vi "StorePAQ.vi"(6 "AverageAction IN":T2, 8 "error in (no error)":errorcluster, 9 "Level":T1, 10 "StoreDatagram":T3 {"Time" format="%#.2f"; "status" format="%x"; "min" format="%.2f"; "max" format="%.2f"; "data" format="%.2f"}, 11 "FAMM in":refnum<class "FAMM.lvclass">) -> (0 "error out":errorcluster, 2 "Next_Level":T2, 3 "FAMM out":refnum<class "FAMM.lvclass">)   [LabVIEW 2020, in "Sgraph_lib_V1.lvlib" / "FAMM.lvclass"]
doc: "Store one element to the PAQ memory"
uses:
  FAMM.lvclass
  controls/MemStoreDatagram.ctl
  controls/typedef_AverageAction.ctl
  controls/typedef_Level.ctl
  FAMM.lvclass/FAMM.ctl
  PAQ-memory.lvclass
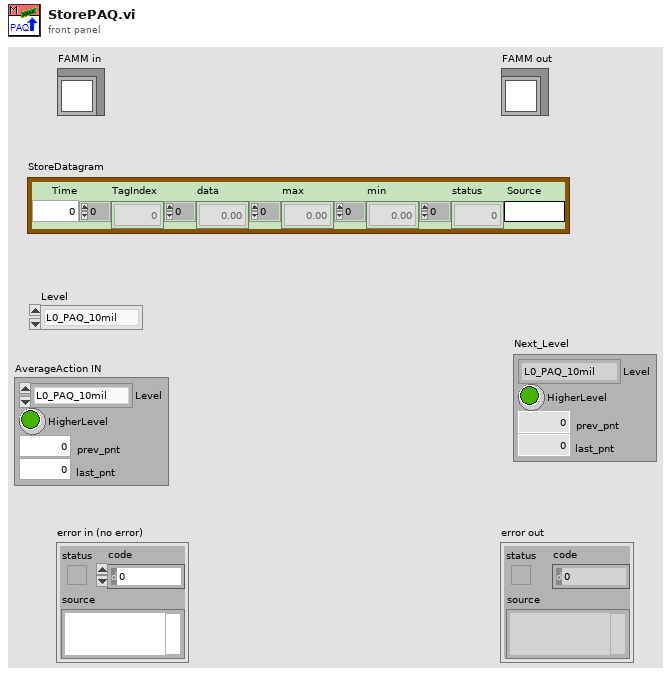
[diagram p1: front panel]
types:
  T1 = typedef "Sgraph_lib_V1.lvlib/FAMM.lvclass/typedef_Level.ctl" = enum16{"L0_PAQ_10mil", "L0_PAQ_100mil", "L1_PAQ_100mil", "L2_PAQ_1sec", "L3_PAQ_10sec", "L4_PAQ_1min", "L5_PAQ_10min", "L6_PAQ_2hr", "L7_PAQ_1day", "L8_PAQ_1wk", "L1_PAQ_1sec", "L2_PAQ_10sec", "L3_PAQ_1min", "L4_PAQ_10min", "L5_PAQ_2hr", "L6_PAQ_1day", "L7_PAQ_1wk", "L0_PAQ_1sec", "L1_PAQ_10sec", "L2_PAQ_1min", "L3_PAQ_10min", "L4_PAQ_2hr", "L5_PAQ_1day", "L6_PAQ_1wk", "L0_PAQ_10sec", "L1_PAQ_1min", "L2_PAQ_10min", "L3_PAQ_2hr", "L4_PAQ_1day", "L5_PAQ_1wk"}
  T2 = typedef "Sgraph_lib_V1.lvlib/FAMM.lvclass/typedef_AverageAction.ctl" = cluster{"Level":T1, "HigherLevel":bool, "prev_pnt":i32, "last_pnt":i32}
  T3 = typedef "Sgraph_lib_V1.lvlib/FAMM.lvclass/MemStoreDatagram.ctl" = cluster{"Time":dbl, "TagIndex":i32[], "data":dbl[], "max":dbl[], "min":dbl[], "status":u32[], "Source":string}
  T4 = cluster{"TAGs":i32[], "prev_pnt":i32, "last_pnt":i32}
  T5 = typedef "Sgraph_lib_V1.lvlib/FAMM.lvclass/FAMM-attributes.ctl" = cluster{"FAMM_PAQ_Layers":i32, "FAMM_PAQ_resolution":dbl, "PAQ_TAGs":string[], "WAQ_TAGs":string[], "EAQ_TAGs":string[], "All_TAGs":string[], "PAQtagProps":T6[], "WAQtagProps":T6[], "EAQtagProps":T6[], "DBAL_class":refnum<data-value>, "PAQ_memory":refnum<data-value>[], "PAQupdates":timestamp[], "FAMM_Size":cluster{"other":i32, "1day":i32, "1week":i32}, "DatabaseFileExtention":string, "DatabaseSaveRate":dbl, "Database_path":path, "DBAL-Queue":refnum<queue>, "OS_name":string, "ini-file":string, "data-retention(days)":dbl}
  T6 = typedef "Sgraph_lib_V1.lvlib/typedef_com_TagProp.ctl" = cluster{"Description":string, "EngUnits":string, "RangeH":dbl, "RangeL":dbl, "Resolution":i32, "Obsolete":bool, "ChangeDate":timestamp, "ChangeSource":string, "ChangeReason":string, "TagFunc":u32}
  T7 = cluster{"Time":dbl, "data":dbl[], "max":dbl[], "min":dbl[], "status":u32[]}
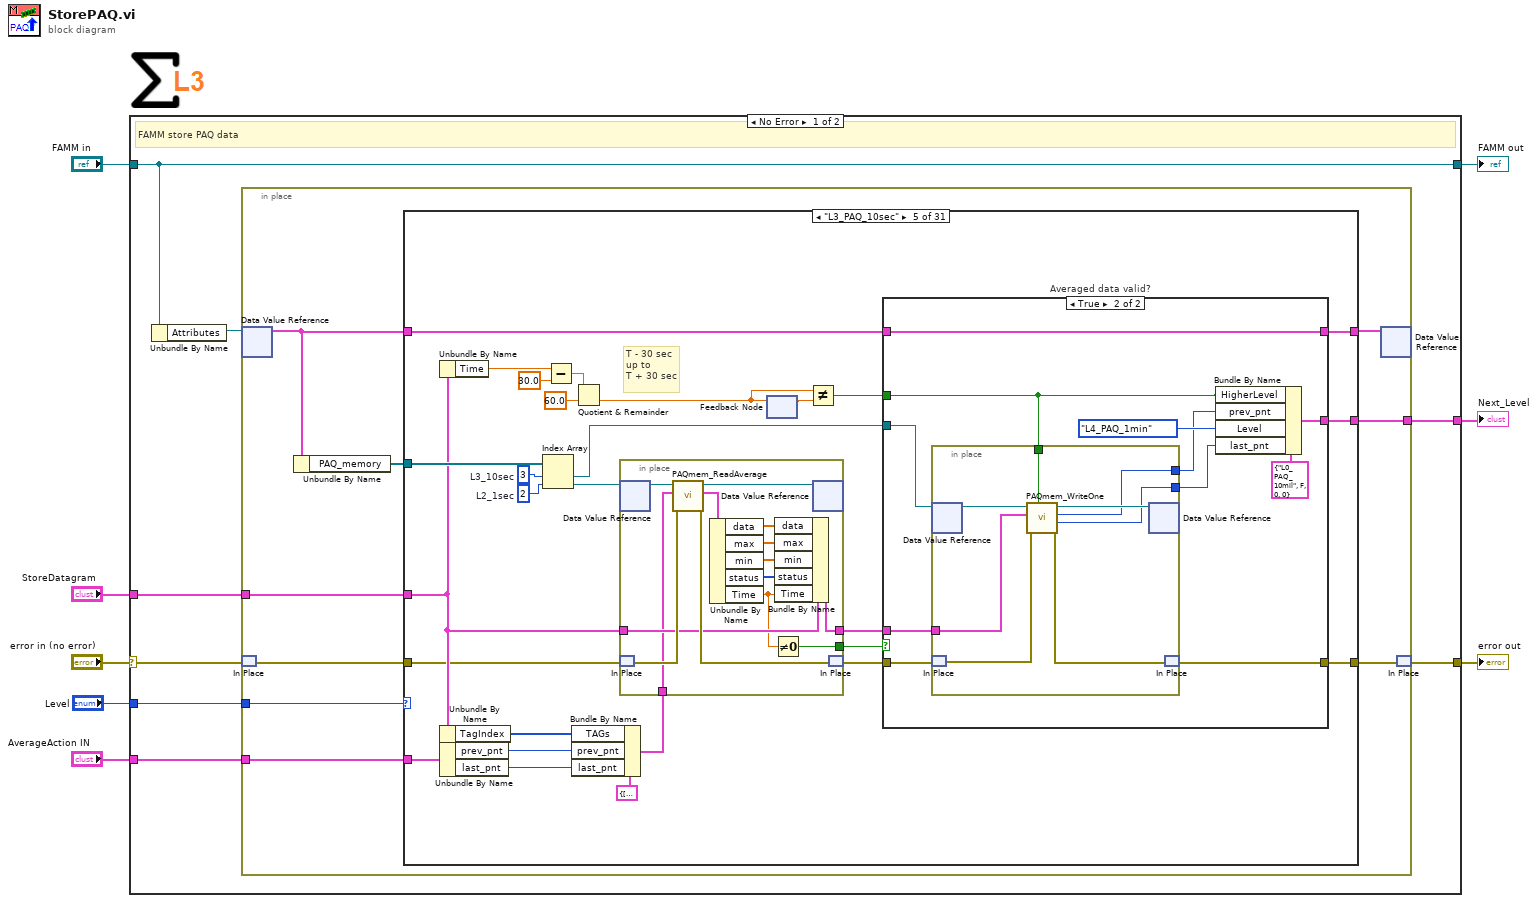
[diagram p0: block diagram]
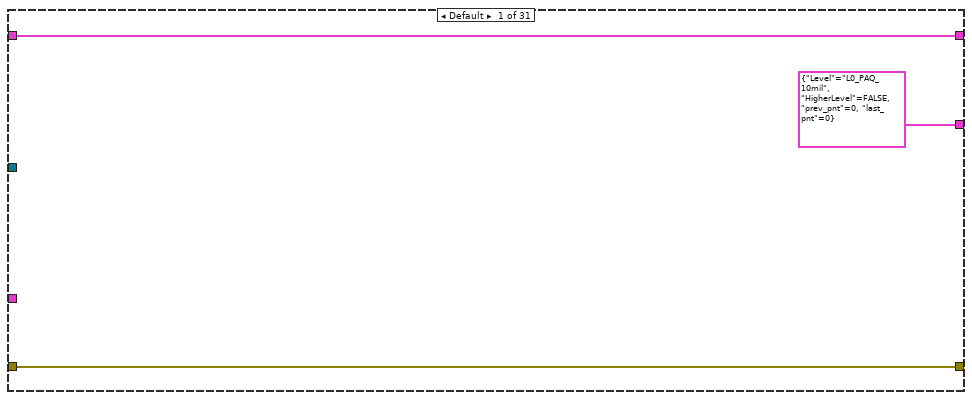
[diagram p2: hidden frame]
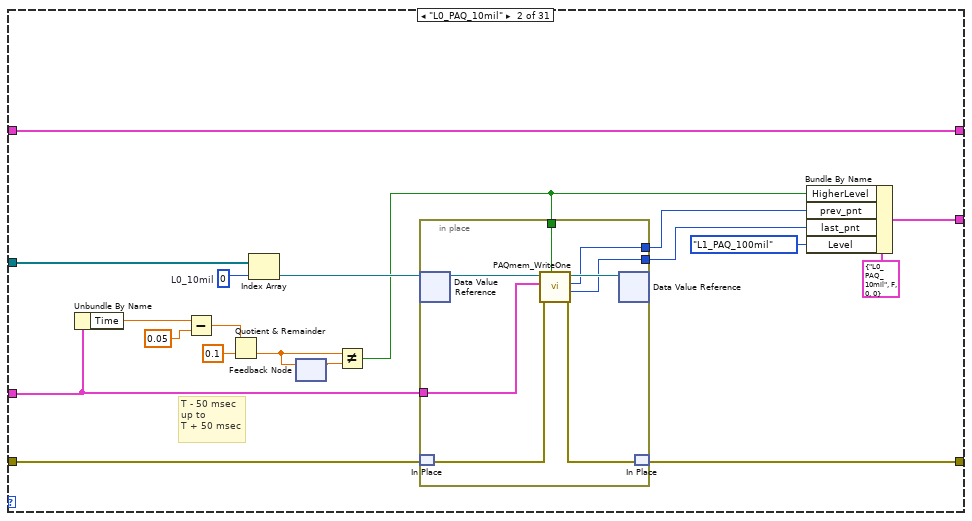
[diagram p3: hidden frame]
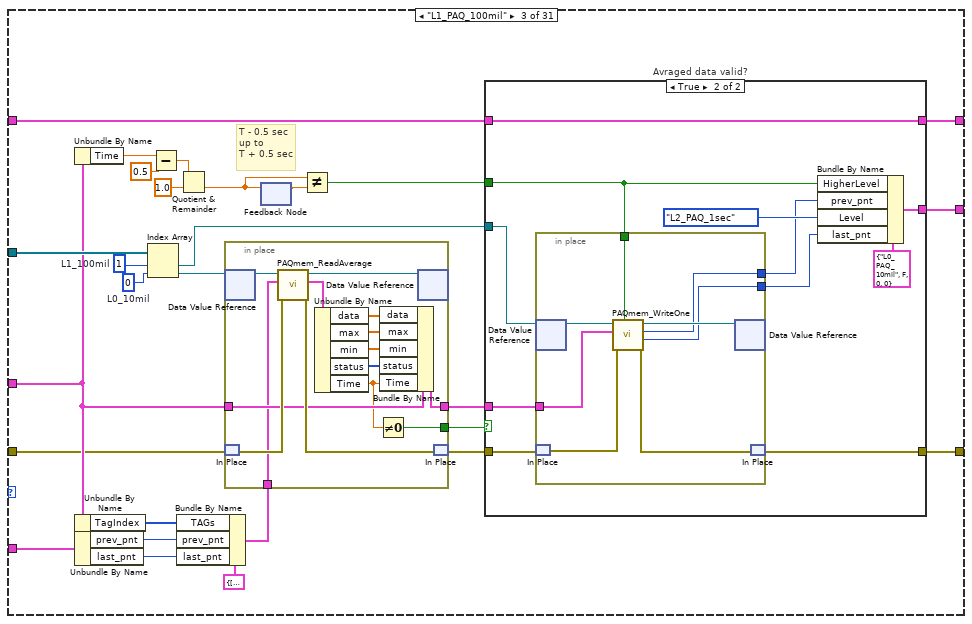
[diagram p4: hidden frame]
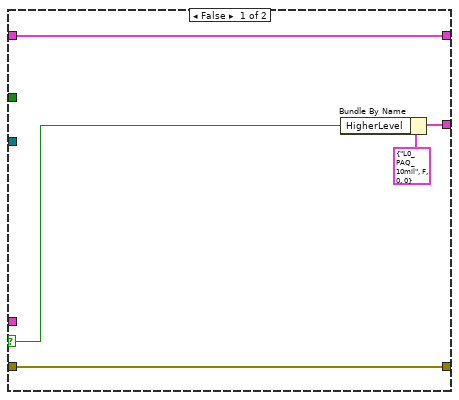
[diagram p5: hidden frame]
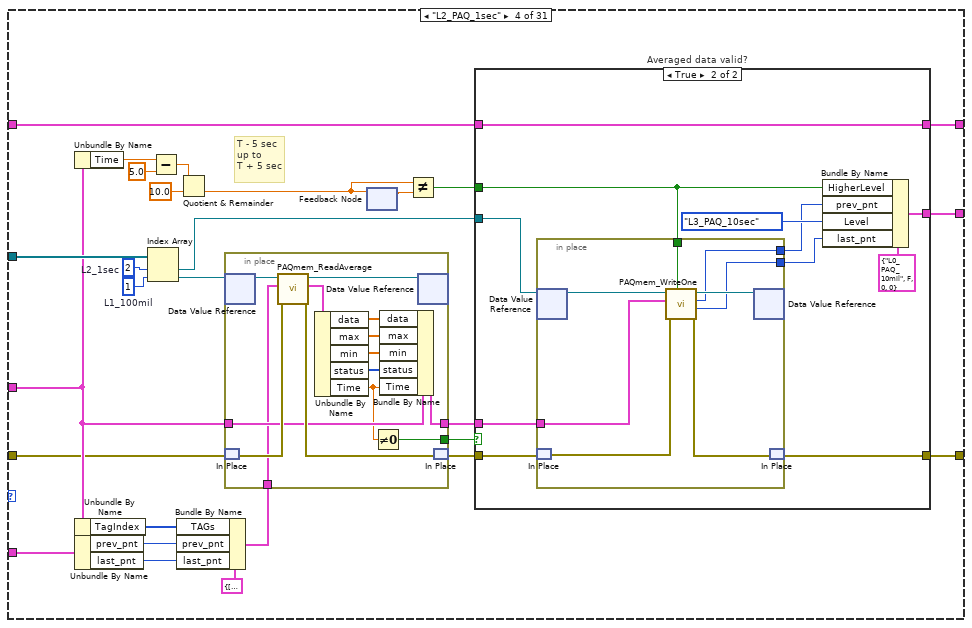
[diagram p6: hidden frame]
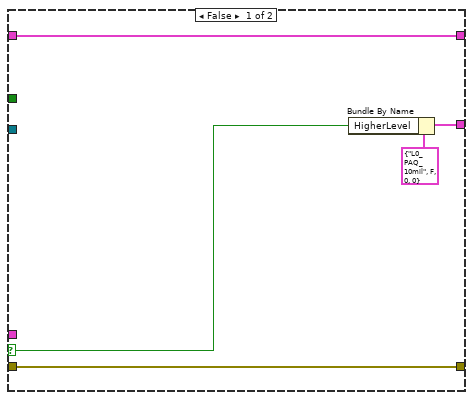
[diagram p7: hidden frame]
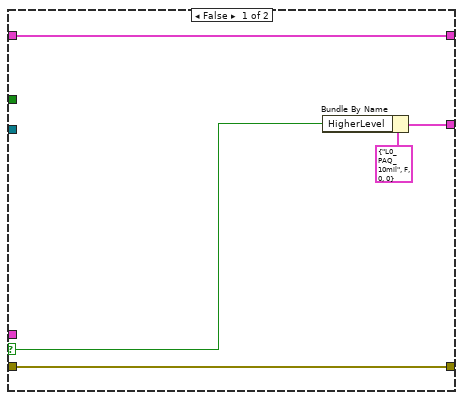
[diagram p8: hidden frame]
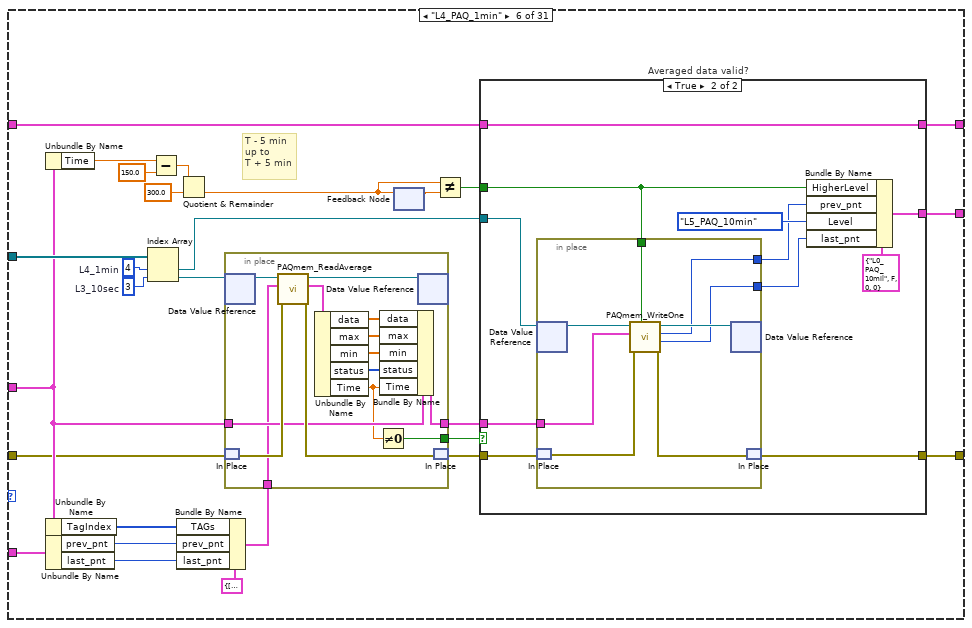
[diagram p9: hidden frame]
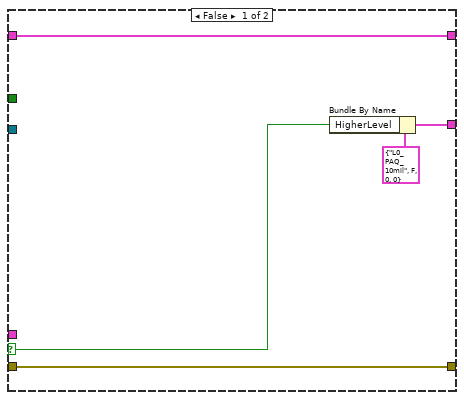
[diagram p10: hidden frame]
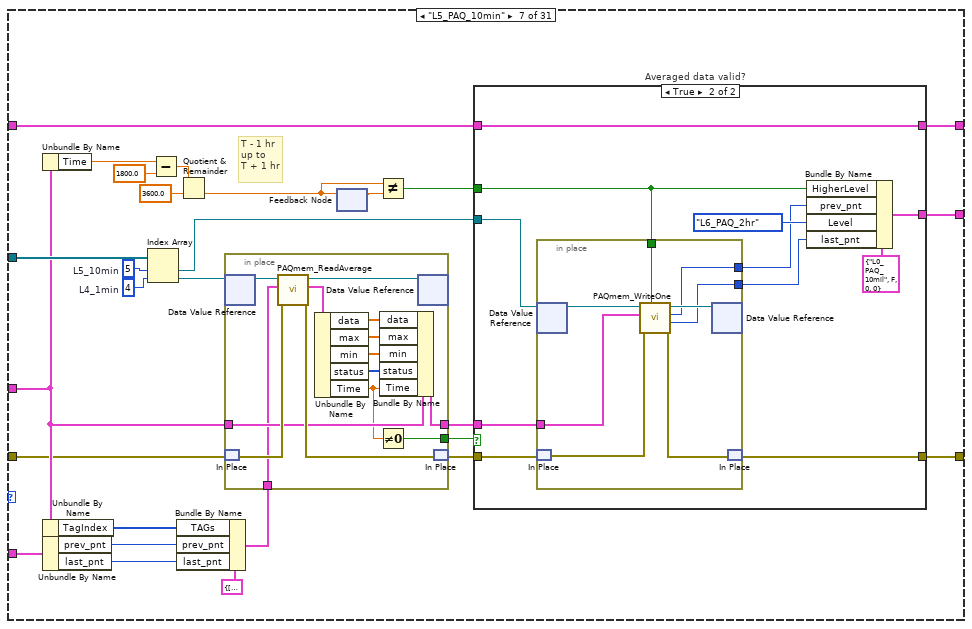
[diagram p11: hidden frame]
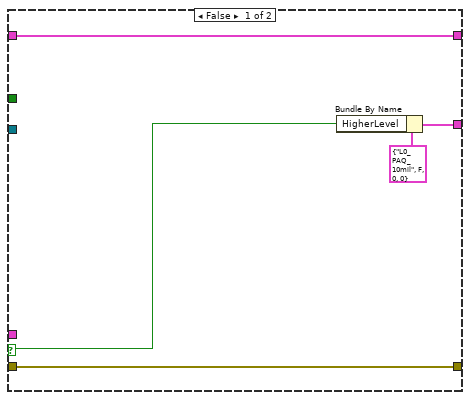
[diagram p12: hidden frame]
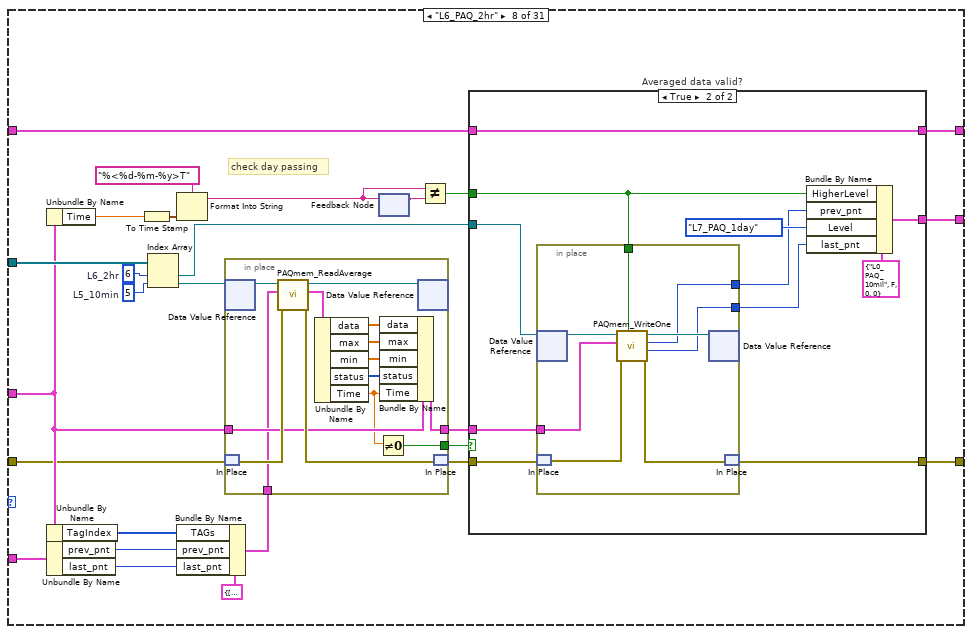
[diagram p13: hidden frame]
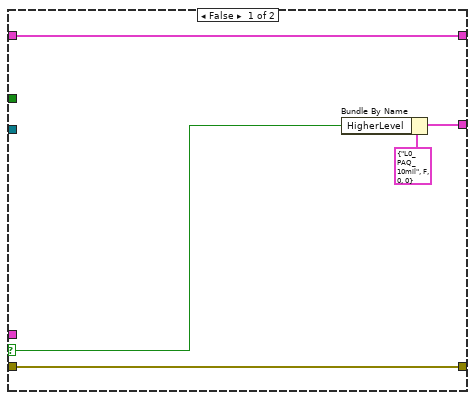
[diagram p14: hidden frame]
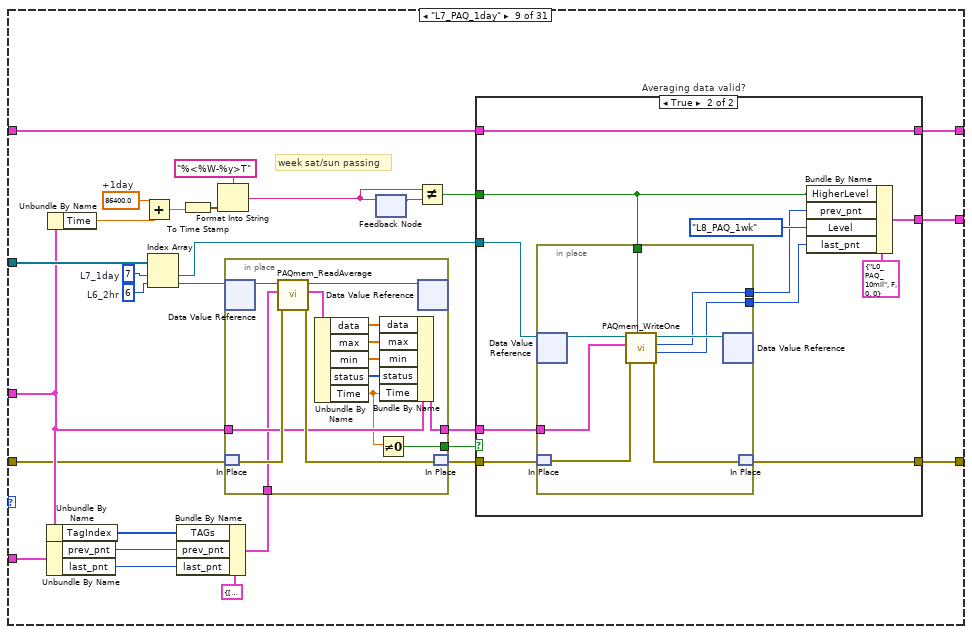
[diagram p15: hidden frame]
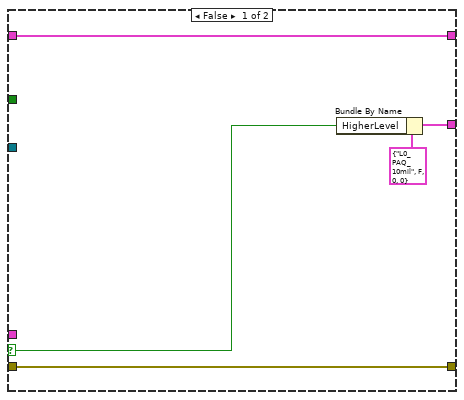
[diagram p16: hidden frame]
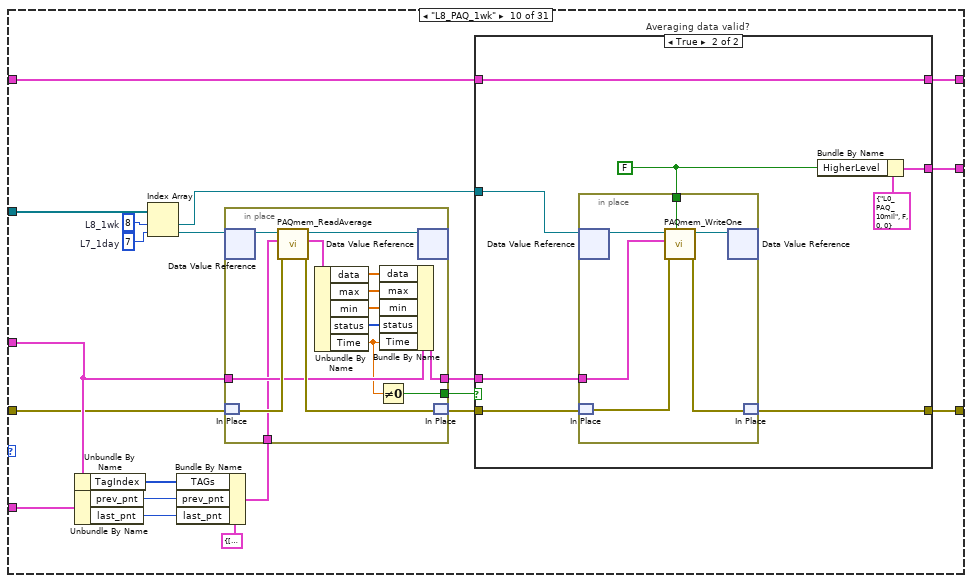
[diagram p17: hidden frame]
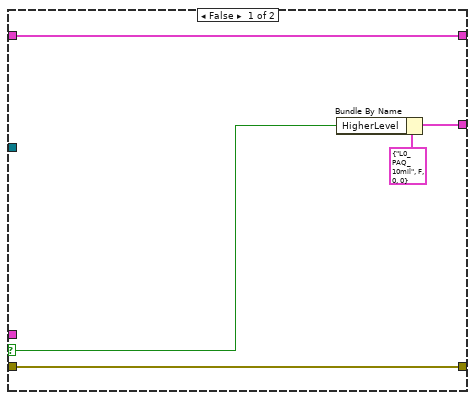
[diagram p18: hidden frame]
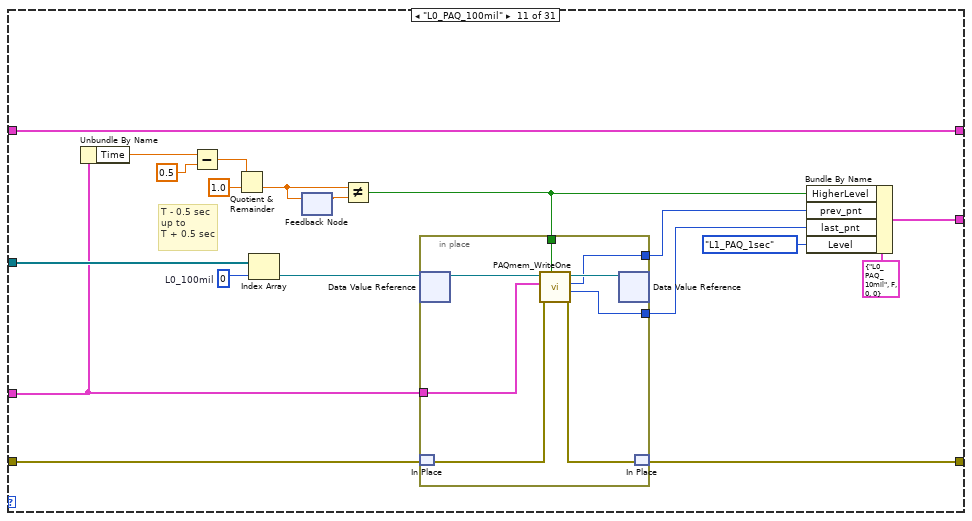
[diagram p19: hidden frame]
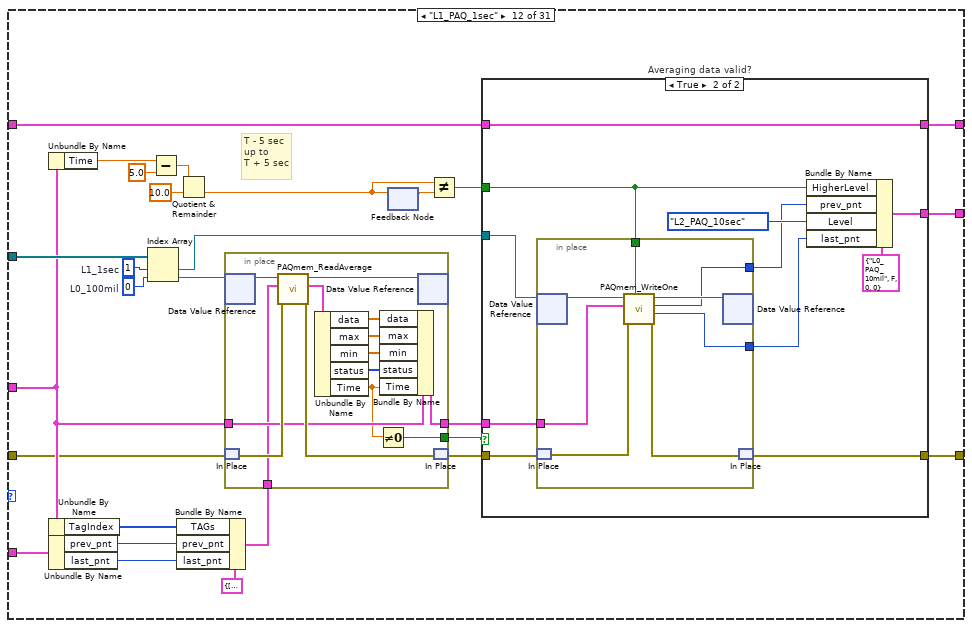
[diagram p20: hidden frame]
diagram:
  n1 = case shown="No Error" "error in (no error)" {
    selector: "error in (no error)" -> [w16 w1779]
    tunnel: [w15 w1779] -> w7
    tunnel: [w10 w1778] -> w5
    tunnel: "FAMM in" -> [w10 w1778]
    tunnel: "StoreDatagram" -> [w14 _]
    tunnel: [w13 _] -> w3
    tunnel: "AverageAction IN" -> [w12 _]
    tunnel: "Level" -> [w11 _]
    frame No Error {
      # "FAMM store PAQ data"
      n2 = Unbundle By Name(w10) -> ("Attributes"=w9:refnum<data-value>)
      n3 = in-place {
        in-place-border: w14 -> [w22]
        in-place-border: [w20] -> w13
        in-place-border: w12 -> [w18]
        in-place-border: w11 -> [w17]
        n4 = in-place-dvr #1(w9) -> (w19:T5)  [unwired: 1 out]
        n5 = in-place-match #2(w16) -> (w24:errorcluster)
        n6 = Unbundle By Name(w19) -> ("PAQ_memory"=w21:refnum<data-value>[])
        n7 = case shown="\"L3_PAQ_10sec\"" w17 {
          tunnel: w19 -> [w28 w31 w57 w144 w209 w274 w339 w403 w469 w527 w564 w614 w679 w743 w808 w872 w938 w996 w1034 w1083 w1148 w1213 w1277 w1343 w1401 w1440 w1488 w1553 w1617 w1683 w1741]
          tunnel: [w28 w31 w79 w143 w208 w273 w338 w402 w468 w526 w564 w613 w678 w742 w807 w871 w937 w995 w1034 w1082 w1147 w1212 w1276 w1342 w1400 w1440 w1487 w1552 w1616 w1682 w1740] -> w25
          tunnel: w24 -> [w27 w47 w56 w132 w197 w262 w327 w395 w461 w519 w582 w602 w667 w731 w796 w864 w930 w988 w1051 w1071 w1136 w1201 w1269 w1335 w1393 w1456 w1476 w1541 w1609 w1675 w1733]
          tunnel: [w27 w46 w82 w147 w212 w277 w342 w406 w472 w530 w581 w617 w682 w746 w811 w875 w941 w999 w1050 w1086 w1151 w1216 w1280 w1346 w1404 w1455 w1491 w1556 w1620 w1686 w1744] -> w23
          tunnel: w22 -> [_ w36 w71 w133 w198 w263 w328 w396 w462 w520 w570 w603 w668 w732 w797 w865 w931 w989 w1039 w1072 w1137 w1202 w1270 w1336 w1394 w1444 w1477 w1542 w1610 w1676 w1734]
          tunnel: w21 -> [_ w45 w81 w146 w211 w276 w341 w405 w471 w529 w580 w616 w681 w745 w810 w874 w940 w998 w1049 w1085 w1150 w1215 w1279 w1345 w1403 w1454 w1490 w1555 w1619 w1685 w1743]
          tunnel: [T2 {"Level"=enum."L0_PAQ_10mil", "HigherLevel"=FALSE, "prev_pnt"=0, "last_pnt"=0} ("AverageAction") w29 w80 w145 w210 w275 w340 w404 w470 w528 w577 w615 w680 w744 w809 w873 w939 w997 w1046 w1084 w1149 w1214 w1278 w1344 w1402 w1451 w1489 w1554 w1618 w1684 w1742] -> w20
          tunnel: w18 -> [_ _ w74 w138 w203 w268 w333 w401 w467 w525 _ w608 w673 w737 w802 w870 w936 w994 _ w1077 w1142 w1207 w1275 w1341 w1399 _ w1482 w1547 w1615 w1681 w1739]
          frame Default {
          }
          frame "L0_PAQ_10mil" {
            w34 = 0  # L0_10mil
            # "T - 50 msec\nup to\nT + 50 msec"
            n8 = Unbundle By Name(w36) -> ("Time"=w41:dbl)
            n9 = Subtract(x=w41, y=0.05) -> (x-y=w39:dbl)
            n10 = Quotient & Remainder(x=w39, y=0.1) -> (floor(x/y)=w38:dbl)  [unwired: 1 out]
            n11 = Index Array(array=w45, index=w34) -> (element=w44:refnum<data-value>)
            n12 = feedback #3() -> (w37:dbl)  [unwired: 1 in]
            n13 = feedback-in #3(w38) -> ()
            n14 = Not Equal?(x=w38, y=w37) -> (x != y?=w30:bool)
            n15 = in-place {
              in-place-border: w36 -> [w53]
              in-place-border: [w50] -> w33
              in-place-border: w30 -> [w49]
              in-place-border: [w48] -> w32
              n16 = in-place-dvr #4(w44) -> (w55:refnum<class "PAQ-memory.lvclass">)  [unwired: 1 out]
              n17 = in-place-match #5(w47) -> (w52:errorcluster)
              n18 = call "PAQmem_WriteOne.vi"("Carry"=w49, "error in (no error)"=w52, "StoreDatagram"=w53, "PAQ-memory in"=w55) -> ("error out"=w51:errorcluster, "Last"=w50:i32, "Prev"=w48:i32, "PAQ-memory out"=w54:refnum<class "PAQ-memory.lvclass">)  [unwired: 4 in]
              n19 = in-place-dvr #4(w54) -> ()  [unwired: 2 out]
              n20 = in-place-match #5(w51) -> (w46:errorcluster)
            }
            n21 = Bundle By Name(cluster=T2 {"Level"=enum."L0_PAQ_10mil", "HigherLevel"=FALSE, "prev_pnt"=0, "last_pnt"=0} ("AverageAction"), "HigherLevel"=w30, "prev_pnt"=w32, "last_pnt"=w33, "Level"=typedef_Level."L1_PAQ_100mil") -> (w29:T2)
          }
          frame "L1_PAQ_100mil" {
            w58 = 1  # L1_100mil
            w66 = 0  # L0_10mil
            # "T - 0.5 sec\nup to\nT + 0.5 sec"
            n22 = Unbundle By Name(w71) -> ("Time"=w77:dbl)
            n23 = Unbundle By Name(w71) -> ("TagIndex"=w73:i32[])
            n24 = Unbundle By Name(w74) -> ("prev_pnt"=w62:i32, "last_pnt"=w63:i32)
            n25 = Index Array(array=w81, index #1=w58, index #2=w66) -> (element #1=w68:refnum<data-value>, element #2=w67:refnum<data-value>)
            n26 = Subtract(x=w77, y=0.5) -> (x-y=w75:dbl)
            n27 = Bundle By Name(cluster=T4 {"TAGs"=[], "prev_pnt"=0, "last_pnt"=0} ("ChunkDefinition"), "TAGs"=w73, "prev_pnt"=w62, "last_pnt"=w63) -> (w69:T4)
            n28 = Quotient & Remainder(x=w75, y=1.0) -> (floor(x/y)=w60:dbl)  [unwired: 1 out]
            n29 = in-place {
              in-place-border: w71 -> [w117]
              in-place-border: [w113] -> w65
              in-place-border: w69 -> [w110]
              in-place-border: [w111] -> w64
              n30 = in-place-dvr #6(w67) -> (w120:refnum<class "PAQ-memory.lvclass">)  [unwired: 1 out]
              n31 = in-place-match #7(w56) -> (w119:errorcluster)
              n32 = call "PAQmem_ReadAverage.vi"("error in (no error)"=w119, "ChunkDefinition"=w110, "PAQ-memory in"=w120) -> ("error out"=w118:errorcluster, "Results"=w109:T7, "PAQ-memory out"=w112:refnum<class "PAQ-memory.lvclass">)  [unwired: 6 in]
              n33 = Unbundle By Name(w109) -> ("data"=w108:dbl[], "max"=w116:dbl[], "min"=w115:dbl[], "status"=w114:u32[], "Time"=w107:dbl)
              n34 = Not Equal To 0?(x=w107) -> (x != 0?=w111:bool)
              n35 = Bundle By Name(cluster=w117, "data"=w108, "max"=w116, "min"=w115, "status"=w114, "Time"=w107) -> (w113:T3)
              n36 = in-place-dvr #6(w112) -> ()  [unwired: 2 out]
              n37 = in-place-match #7(w118) -> (w70:errorcluster)
            }
            n38 = feedback #8() -> (w61:dbl)  [unwired: 1 in]
            n39 = feedback-in #8(w60) -> ()
            n40 = Not Equal?(x=w60, y=w61) -> (x != y?=w59:bool)
            n41 = case "Avraged data valid?" shown="True" w64 {
              selector: w64 -> [w84 _]
              tunnel: [w83 w98] -> w82
              tunnel: [w85 w96] -> w80
              tunnel: w57 -> [w87 w88]
              tunnel: [w87 w88] -> w79
              tunnel: w70 -> [w83 w95]
              tunnel: w68 -> [_ w94]
              tunnel: w65 -> [_ w93]
              tunnel: w59 -> [_ w90]
              frame False {
                n42 = Bundle By Name(cluster=T2 {"Level"=enum."L0_PAQ_10mil", "HigherLevel"=FALSE, "prev_pnt"=0, "last_pnt"=0} ("AverageAction"), "HigherLevel"=w84) -> (w85:T2)
              }
              frame True {
                n43 = in-place {
                  in-place-border: w93 -> [w101]
                  in-place-border: [w104] -> w91
                  in-place-border: w90 -> [w100]
                  in-place-border: [w99] -> w89
                  n44 = in-place-dvr #9(w94) -> (w103:refnum<class "PAQ-memory.lvclass">)  [unwired: 1 out]
                  n45 = in-place-match #10(w95) -> (w102:errorcluster)
                  n46 = call "PAQmem_WriteOne.vi"("Carry"=w100, "error in (no error)"=w102, "StoreDatagram"=w101, "PAQ-memory in"=w103) -> ("error out"=w105:errorcluster, "Last"=w104:i32, "Prev"=w99:i32, "PAQ-memory out"=w106:refnum<class "PAQ-memory.lvclass">)  [unwired: 4 in]
                  n47 = in-place-dvr #9(w106) -> ()  [unwired: 2 out]
                  n48 = in-place-match #10(w105) -> (w98:errorcluster)
                }
                n49 = Bundle By Name(cluster=T2 {"Level"=enum."L0_PAQ_10mil", "HigherLevel"=FALSE, "prev_pnt"=0, "last_pnt"=0} ("AverageAction"), "HigherLevel"=w90, "prev_pnt"=w89, "Level"=typedef_Level."L2_PAQ_1sec", "last_pnt"=w91) -> (w96:T2)
              }
            }
          }
          frame "L2_PAQ_1sec" {
            w125 = 2  # L2_1sec
            w127 = 1  # L1_100mil
            # "T - 5 sec\nup to\nT + 5 sec"
            n50 = Unbundle By Name(w133) -> ("Time"=w141:dbl)
            n51 = Unbundle By Name(w133) -> ("TagIndex"=w137:i32[])
            n52 = Unbundle By Name(w138) -> ("prev_pnt"=w135:i32, "last_pnt"=w134:i32)
            n53 = Index Array(array=w146, index #1=w125, index #2=w127) -> (element #1=w129:refnum<data-value>, element #2=w128:refnum<data-value>)
            n54 = Subtract(x=w141, y=5.0) -> (x-y=w139:dbl)
            n55 = Bundle By Name(cluster=T4 {"TAGs"=[], "prev_pnt"=0, "last_pnt"=0} ("ChunkDefinition"), "TAGs"=w137, "prev_pnt"=w135, "last_pnt"=w134) -> (w130:T4)
            n56 = Quotient & Remainder(x=w139, y=10.0) -> (floor(x/y)=w122:dbl)  [unwired: 1 out]
            n57 = in-place {
              in-place-border: w133 -> [w181]
              in-place-border: [w176] -> w126
              in-place-border: w130 -> [w174]
              in-place-border: [w172] -> w124
              n58 = in-place-dvr #11(w128) -> (w184:refnum<class "PAQ-memory.lvclass">)  [unwired: 1 out]
              n59 = in-place-match #12(w132) -> (w183:errorcluster)
              n60 = call "PAQmem_ReadAverage.vi"("error in (no error)"=w183, "ChunkDefinition"=w174, "PAQ-memory in"=w184) -> ("error out"=w182:errorcluster, "Results"=w185:T7, "PAQ-memory out"=w175:refnum<class "PAQ-memory.lvclass">)  [unwired: 6 in]
              n61 = Unbundle By Name(w185) -> ("data"=w180:dbl[], "max"=w179:dbl[], "min"=w178:dbl[], "status"=w177:u32[], "Time"=w173:dbl)
              n62 = Not Equal To 0?(x=w173) -> (x != 0?=w172:bool)
              n63 = Bundle By Name(cluster=w181, "data"=w180, "max"=w179, "min"=w178, "status"=w177, "Time"=w173) -> (w176:T3)
              n64 = in-place-dvr #11(w175) -> ()  [unwired: 2 out]
              n65 = in-place-match #12(w182) -> (w131:errorcluster)
            }
            n66 = feedback #13() -> (w123:dbl)  [unwired: 1 in]
            n67 = feedback-in #13(w122) -> ()
            n68 = Not Equal?(x=w122, y=w123) -> (x != y?=w121:bool)
            n69 = case "Averaged data valid?" shown="True" w124 {
              selector: w124 -> [w151 _]
              tunnel: [w150 w163] -> w147
              tunnel: [w148 w161] -> w145
              tunnel: w144 -> [w149 w153]
              tunnel: [w149 w153] -> w143
              tunnel: w131 -> [w150 w160]
              tunnel: w129 -> [_ w159]
              tunnel: w126 -> [_ w158]
              tunnel: w121 -> [_ w155]
              frame False {
                n70 = Bundle By Name(cluster=T2 {"Level"=enum."L0_PAQ_10mil", "HigherLevel"=FALSE, "prev_pnt"=0, "last_pnt"=0} ("AverageAction"), "HigherLevel"=w151) -> (w148:T2)
              }
              frame True {
                n71 = in-place {
                  in-place-border: w158 -> [w166]
                  in-place-border: [w169] -> w156
                  in-place-border: w155 -> [w165]
                  in-place-border: [w164] -> w154
                  n72 = in-place-dvr #14(w159) -> (w168:refnum<class "PAQ-memory.lvclass">)  [unwired: 1 out]
                  n73 = in-place-match #15(w160) -> (w167:errorcluster)
                  n74 = call "PAQmem_WriteOne.vi"("Carry"=w165, "error in (no error)"=w167, "StoreDatagram"=w166, "PAQ-memory in"=w168) -> ("error out"=w170:errorcluster, "Last"=w169:i32, "Prev"=w164:i32, "PAQ-memory out"=w171:refnum<class "PAQ-memory.lvclass">)  [unwired: 4 in]
                  n75 = in-place-dvr #14(w171) -> ()  [unwired: 2 out]
                  n76 = in-place-match #15(w170) -> (w163:errorcluster)
                }
                n77 = Bundle By Name(cluster=T2 {"Level"=enum."L0_PAQ_10mil", "HigherLevel"=FALSE, "prev_pnt"=0, "last_pnt"=0} ("AverageAction"), "HigherLevel"=w155, "prev_pnt"=w154, "Level"=typedef_Level."L3_PAQ_10sec", "last_pnt"=w156) -> (w161:T2)
              }
            }
          }
          frame "L3_PAQ_10sec" {
            w190 = 3  # L3_10sec
            w192 = 2  # L2_1sec
            # "T - 30 sec\nup to\nT + 30 sec"
            n78 = Unbundle By Name(w198) -> ("Time"=w206:dbl)
            n79 = Unbundle By Name(w198) -> ("TagIndex"=w202:i32[])
            n80 = Unbundle By Name(w203) -> ("prev_pnt"=w200:i32, "last_pnt"=w199:i32)
            n81 = Index Array(array=w211, index #1=w190, index #2=w192) -> (element #1=w194:refnum<data-value>, element #2=w193:refnum<data-value>)
            n82 = Subtract(x=w206, y=30.0) -> (x-y=w204:dbl)
            n83 = Bundle By Name(cluster=T4 {"TAGs"=[], "prev_pnt"=0, "last_pnt"=0} ("ChunkDefinition"), "TAGs"=w202, "prev_pnt"=w200, "last_pnt"=w199) -> (w195:T4)
            n84 = Quotient & Remainder(x=w204, y=60.0) -> (floor(x/y)=w187:dbl)  [unwired: 1 out]
            n85 = in-place {
              in-place-border: w198 -> [w246]
              in-place-border: [w241] -> w191
              in-place-border: w195 -> [w239]
              in-place-border: [w237] -> w189
              n86 = in-place-dvr #16(w193) -> (w249:refnum<class "PAQ-memory.lvclass">)  [unwired: 1 out]
              n87 = in-place-match #17(w197) -> (w248:errorcluster)
              n88 = call "PAQmem_ReadAverage.vi"("error in (no error)"=w248, "ChunkDefinition"=w239, "PAQ-memory in"=w249) -> ("error out"=w247:errorcluster, "Results"=w250:T7, "PAQ-memory out"=w240:refnum<class "PAQ-memory.lvclass">)  [unwired: 6 in]
              n89 = Unbundle By Name(w250) -> ("data"=w245:dbl[], "max"=w244:dbl[], "min"=w243:dbl[], "status"=w242:u32[], "Time"=w238:dbl)
              n90 = Not Equal To 0?(x=w238) -> (x != 0?=w237:bool)
              n91 = Bundle By Name(cluster=w246, "data"=w245, "max"=w244, "min"=w243, "status"=w242, "Time"=w238) -> (w241:T3)
              n92 = in-place-dvr #16(w240) -> ()  [unwired: 2 out]
              n93 = in-place-match #17(w247) -> (w196:errorcluster)
            }
            n94 = feedback #18() -> (w188:dbl)  [unwired: 1 in]
            n95 = feedback-in #18(w187) -> ()
            n96 = Not Equal?(x=w187, y=w188) -> (x != y?=w186:bool)
            n97 = case "Averaged data valid?" shown="True" w189 {
              selector: w189 -> [w216 _]
              tunnel: [w214 w228] -> w212
              tunnel: [w215 w226] -> w210
              tunnel: w209 -> [w213 w218]
              tunnel: [w213 w218] -> w208
              tunnel: w196 -> [w214 w225]
              tunnel: w194 -> [_ w224]
              tunnel: w191 -> [_ w223]
              tunnel: w186 -> [_ w219]
              frame False {
                n98 = Bundle By Name(cluster=T2 {"Level"=enum."L0_PAQ_10mil", "HigherLevel"=FALSE, "prev_pnt"=0, "last_pnt"=0} ("AverageAction"), "HigherLevel"=w216) -> (w215:T2)
              }
              frame True {
                n99 = in-place {
                  in-place-border: w223 -> [w231]
                  in-place-border: [w234] -> w221
                  in-place-border: [w230] -> w220
                  in-place-border: w219 -> [w229]
                  n100 = in-place-dvr #19(w224) -> (w233:refnum<class "PAQ-memory.lvclass">)  [unwired: 1 out]
                  n101 = in-place-match #20(w225) -> (w232:errorcluster)
                  n102 = call "PAQmem_WriteOne.vi"("Carry"=w229, "error in (no error)"=w232, "StoreDatagram"=w231, "PAQ-memory in"=w233) -> ("error out"=w235:errorcluster, "Last"=w234:i32, "Prev"=w230:i32, "PAQ-memory out"=w236:refnum<class "PAQ-memory.lvclass">)  [unwired: 4 in]
                  n103 = in-place-dvr #19(w236) -> ()  [unwired: 2 out]
                  n104 = in-place-match #20(w235) -> (w228:errorcluster)
                }
                n105 = Bundle By Name(cluster=T2 {"Level"=enum."L0_PAQ_10mil", "HigherLevel"=FALSE, "prev_pnt"=0, "last_pnt"=0} ("AverageAction"), "HigherLevel"=w219, "prev_pnt"=w220, "Level"=typedef_Level."L4_PAQ_1min", "last_pnt"=w221) -> (w226:T2)
              }
            }
          }
          frame "L4_PAQ_1min" {
            w255 = 4  # L4_1min
            w257 = 3  # L3_10sec
            # "T - 5 min\nup to\nT + 5 min"
            n106 = Unbundle By Name(w263) -> ("Time"=w271:dbl)
            n107 = Unbundle By Name(w263) -> ("TagIndex"=w267:i32[])
            n108 = Unbundle By Name(w268) -> ("prev_pnt"=w265:i32, "last_pnt"=w264:i32)
            n109 = Index Array(array=w276, index #1=w255, index #2=w257) -> (element #1=w259:refnum<data-value>, element #2=w258:refnum<data-value>)
            n110 = Subtract(x=w271, y=150.0) -> (x-y=w269:dbl)
            n111 = Bundle By Name(cluster=T4 {"TAGs"=[], "prev_pnt"=0, "last_pnt"=0} ("ChunkDefinition"), "TAGs"=w267, "prev_pnt"=w265, "last_pnt"=w264) -> (w260:T4)
            n112 = Quotient & Remainder(x=w269, y=300.0) -> (floor(x/y)=w252:dbl)  [unwired: 1 out]
            n113 = in-place {
              in-place-border: w263 -> [w311]
              in-place-border: [w306] -> w256
              in-place-border: w260 -> [w304]
              in-place-border: [w302] -> w254
              n114 = in-place-dvr #21(w258) -> (w314:refnum<class "PAQ-memory.lvclass">)  [unwired: 1 out]
              n115 = in-place-match #22(w262) -> (w313:errorcluster)
              n116 = call "PAQmem_ReadAverage.vi"("error in (no error)"=w313, "ChunkDefinition"=w304, "PAQ-memory in"=w314) -> ("error out"=w312:errorcluster, "Results"=w315:T7, "PAQ-memory out"=w305:refnum<class "PAQ-memory.lvclass">)  [unwired: 6 in]
              n117 = Unbundle By Name(w315) -> ("data"=w310:dbl[], "max"=w309:dbl[], "min"=w308:dbl[], "status"=w307:u32[], "Time"=w303:dbl)
              n118 = Not Equal To 0?(x=w303) -> (x != 0?=w302:bool)
              n119 = Bundle By Name(cluster=w311, "data"=w310, "max"=w309, "min"=w308, "status"=w307, "Time"=w303) -> (w306:T3)
              n120 = in-place-dvr #21(w305) -> ()  [unwired: 2 out]
              n121 = in-place-match #22(w312) -> (w261:errorcluster)
            }
            n122 = feedback #23() -> (w253:dbl)  [unwired: 1 in]
            n123 = feedback-in #23(w252) -> ()
            n124 = Not Equal?(x=w252, y=w253) -> (x != y?=w251:bool)
            n125 = case "Averaged data valid?" shown="True" w254 {
              selector: w254 -> [w280 _]
              tunnel: [w279 w293] -> w277
              tunnel: [w281 w291] -> w275
              tunnel: w274 -> [w278 w283]
              tunnel: [w278 w283] -> w273
              tunnel: w261 -> [w279 w290]
              tunnel: w259 -> [_ w289]
              tunnel: w256 -> [_ w288]
              tunnel: w251 -> [_ w285]
              frame False {
                n126 = Bundle By Name(cluster=T2 {"Level"=enum."L0_PAQ_10mil", "HigherLevel"=FALSE, "prev_pnt"=0, "last_pnt"=0} ("AverageAction"), "HigherLevel"=w280) -> (w281:T2)
              }
              frame True {
                n127 = in-place {
                  in-place-border: w288 -> [w296]
                  in-place-border: [w299] -> w286
                  in-place-border: w285 -> [w295]
                  in-place-border: [w294] -> w284
                  n128 = in-place-dvr #24(w289) -> (w298:refnum<class "PAQ-memory.lvclass">)  [unwired: 1 out]
                  n129 = in-place-match #25(w290) -> (w297:errorcluster)
                  n130 = call "PAQmem_WriteOne.vi"("Carry"=w295, "error in (no error)"=w297, "StoreDatagram"=w296, "PAQ-memory in"=w298) -> ("error out"=w300:errorcluster, "Last"=w299:i32, "Prev"=w294:i32, "PAQ-memory out"=w301:refnum<class "PAQ-memory.lvclass">)  [unwired: 4 in]
                  n131 = in-place-dvr #24(w301) -> ()  [unwired: 2 out]
                  n132 = in-place-match #25(w300) -> (w293:errorcluster)
                }
                n133 = Bundle By Name(cluster=T2 {"Level"=enum."L0_PAQ_10mil", "HigherLevel"=FALSE, "prev_pnt"=0, "last_pnt"=0} ("AverageAction"), "HigherLevel"=w285, "prev_pnt"=w284, "Level"=typedef_Level."L5_PAQ_10min", "last_pnt"=w286) -> (w291:T2)
              }
            }
          }
          frame "L5_PAQ_10min" {
            w320 = 5  # L5_10min
            w322 = 4  # L4_1min
            # "T - 1 hr\nup to\nT + 1 hr"
            n134 = Unbundle By Name(w328) -> ("Time"=w336:dbl)
            n135 = Unbundle By Name(w328) -> ("TagIndex"=w332:i32[])
            n136 = Unbundle By Name(w333) -> ("prev_pnt"=w330:i32, "last_pnt"=w329:i32)
            n137 = Index Array(array=w341, index #1=w320, index #2=w322) -> (element #1=w324:refnum<data-value>, element #2=w323:refnum<data-value>)
            n138 = Subtract(x=w336, y=1800.0) -> (x-y=w334:dbl)
            n139 = Bundle By Name(cluster=T4 {"TAGs"=[], "prev_pnt"=0, "last_pnt"=0} ("ChunkDefinition"), "TAGs"=w332, "prev_pnt"=w330, "last_pnt"=w329) -> (w325:T4)
            n140 = Quotient & Remainder(x=w334, y=3600.0) -> (floor(x/y)=w317:dbl)  [unwired: 1 out]
            n141 = in-place {
              in-place-border: w328 -> [w376]
              in-place-border: [w371] -> w321
              in-place-border: w325 -> [w369]
              in-place-border: [w367] -> w319
              n142 = in-place-dvr #26(w323) -> (w379:refnum<class "PAQ-memory.lvclass">)  [unwired: 1 out]
              n143 = in-place-match #27(w327) -> (w378:errorcluster)
              n144 = call "PAQmem_ReadAverage.vi"("error in (no error)"=w378, "ChunkDefinition"=w369, "PAQ-memory in"=w379) -> ("error out"=w377:errorcluster, "Results"=w380:T7, "PAQ-memory out"=w370:refnum<class "PAQ-memory.lvclass">)  [unwired: 6 in]
              n145 = Unbundle By Name(w380) -> ("data"=w375:dbl[], "max"=w374:dbl[], "min"=w373:dbl[], "status"=w372:u32[], "Time"=w368:dbl)
              n146 = Not Equal To 0?(x=w368) -> (x != 0?=w367:bool)
              n147 = Bundle By Name(cluster=w376, "data"=w375, "max"=w374, "min"=w373, "status"=w372, "Time"=w368) -> (w371:T3)
              n148 = in-place-dvr #26(w370) -> ()  [unwired: 2 out]
              n149 = in-place-match #27(w377) -> (w326:errorcluster)
            }
            n150 = feedback #28() -> (w318:dbl)  [unwired: 1 in]
            n151 = feedback-in #28(w317) -> ()
            n152 = Not Equal?(x=w317, y=w318) -> (x != y?=w316:bool)
            n153 = case "Averaged data valid?" shown="True" w319 {
              selector: w319 -> [w344 _]
              tunnel: [w346 w358] -> w342
              tunnel: [w343 w356] -> w340
              tunnel: w339 -> [w347 w350]
              tunnel: [w347 w350] -> w338
              tunnel: w326 -> [w346 w355]
              tunnel: w324 -> [_ w354]
              tunnel: w321 -> [_ w353]
              tunnel: w316 -> [_ w348]
              frame False {
                n154 = Bundle By Name(cluster=T2 {"Level"=enum."L0_PAQ_10mil", "HigherLevel"=FALSE, "prev_pnt"=0, "last_pnt"=0} ("AverageAction"), "HigherLevel"=w344) -> (w343:T2)
              }
              frame True {
                n155 = in-place {
                  in-place-border: w353 -> [w361]
                  in-place-border: [w364] -> w351
                  in-place-border: [w360] -> w349
                  in-place-border: w348 -> [w359]
                  n156 = in-place-dvr #29(w354) -> (w363:refnum<class "PAQ-memory.lvclass">)  [unwired: 1 out]
                  n157 = in-place-match #30(w355) -> (w362:errorcluster)
                  n158 = call "PAQmem_WriteOne.vi"("Carry"=w359, "error in (no error)"=w362, "StoreDatagram"=w361, "PAQ-memory in"=w363) -> ("error out"=w365:errorcluster, "Last"=w364:i32, "Prev"=w360:i32, "PAQ-memory out"=w366:refnum<class "PAQ-memory.lvclass">)  [unwired: 4 in]
                  n159 = in-place-dvr #29(w366) -> ()  [unwired: 2 out]
                  n160 = in-place-match #30(w365) -> (w358:errorcluster)
                }
                n161 = Bundle By Name(cluster=T2 {"Level"=enum."L0_PAQ_10mil", "HigherLevel"=FALSE, "prev_pnt"=0, "last_pnt"=0} ("AverageAction"), "HigherLevel"=w348, "prev_pnt"=w349, "Level"=typedef_Level."L6_PAQ_2hr", "last_pnt"=w351) -> (w356:T2)
              }
            }
          }
          frame "L6_PAQ_2hr" {
            w388 = 6  # L6_2hr
            w390 = 5  # L5_10min
            # "check day passing"
            n162 = Unbundle By Name(w396) -> ("Time"=w387:dbl)
            n163 = Unbundle By Name(w396) -> ("TagIndex"=w400:i32[])
            n164 = Unbundle By Name(w401) -> ("prev_pnt"=w398:i32, "last_pnt"=w397:i32)
            n165 = To Time Stamp(1:w387) -> (0:w386:timestamp)
            n166 = Index Array(array=w405, index #1=w388, index #2=w390) -> (element #1=w392:refnum<data-value>, element #2=w391:refnum<data-value>)
            n167 = Format Into String(format string="%<%d-%m-%y>T", w386) -> (resulting string=w382:string)  [unwired: 2 in, 1 out]
            n168 = Bundle By Name(cluster=T4 {"TAGs"=[], "prev_pnt"=0, "last_pnt"=0} ("ChunkDefinition"), "TAGs"=w400, "prev_pnt"=w398, "last_pnt"=w397) -> (w393:T4)
            n169 = in-place {
              in-place-border: w396 -> [w440]
              in-place-border: [w435] -> w389
              in-place-border: w393 -> [w433]
              in-place-border: [w431] -> w384
              n170 = in-place-dvr #31(w391) -> (w443:refnum<class "PAQ-memory.lvclass">)  [unwired: 1 out]
              n171 = in-place-match #32(w395) -> (w442:errorcluster)
              n172 = call "PAQmem_ReadAverage.vi"("error in (no error)"=w442, "ChunkDefinition"=w433, "PAQ-memory in"=w443) -> ("error out"=w441:errorcluster, "Results"=w444:T7, "PAQ-memory out"=w434:refnum<class "PAQ-memory.lvclass">)  [unwired: 6 in]
              n173 = Unbundle By Name(w444) -> ("data"=w439:dbl[], "max"=w438:dbl[], "min"=w437:dbl[], "status"=w436:u32[], "Time"=w432:dbl)
              n174 = Not Equal To 0?(x=w432) -> (x != 0?=w431:bool)
              n175 = Bundle By Name(cluster=w440, "data"=w439, "max"=w438, "min"=w437, "status"=w436, "Time"=w432) -> (w435:T3)
              n176 = in-place-dvr #31(w434) -> ()  [unwired: 2 out]
              n177 = in-place-match #32(w441) -> (w394:errorcluster)
            }
            n178 = feedback #33() -> (w383:string)  [unwired: 1 in]
            n179 = feedback-in #33(w382) -> ()
            n180 = Not Equal?(x=w382, y=w383) -> (x != y?=w381:bool)
            n181 = case "Averaged data valid?" shown="True" w384 {
              selector: w384 -> [w410 _]
              tunnel: [w407 w422] -> w406
              tunnel: [w409 w420] -> w404
              tunnel: w403 -> [w408 w412]
              tunnel: [w408 w412] -> w402
              tunnel: w394 -> [w407 w419]
              tunnel: w392 -> [_ w418]
              tunnel: w389 -> [_ w417]
              tunnel: w381 -> [_ w413]
              frame False {
                n182 = Bundle By Name(cluster=T2 {"Level"=enum."L0_PAQ_10mil", "HigherLevel"=FALSE, "prev_pnt"=0, "last_pnt"=0} ("AverageAction"), "HigherLevel"=w410) -> (w409:T2)
              }
              frame True {
                n183 = in-place {
                  in-place-border: w417 -> [w425]
                  in-place-border: [w428] -> w415
                  in-place-border: [w424] -> w414
                  in-place-border: w413 -> [w423]
                  n184 = in-place-dvr #34(w418) -> (w427:refnum<class "PAQ-memory.lvclass">)  [unwired: 1 out]
                  n185 = in-place-match #35(w419) -> (w426:errorcluster)
                  n186 = call "PAQmem_WriteOne.vi"("Carry"=w423, "error in (no error)"=w426, "StoreDatagram"=w425, "PAQ-memory in"=w427) -> ("error out"=w429:errorcluster, "Last"=w428:i32, "Prev"=w424:i32, "PAQ-memory out"=w430:refnum<class "PAQ-memory.lvclass">)  [unwired: 4 in]
                  n187 = in-place-dvr #34(w430) -> ()  [unwired: 2 out]
                  n188 = in-place-match #35(w429) -> (w422:errorcluster)
                }
                n189 = Bundle By Name(cluster=T2 {"Level"=enum."L0_PAQ_10mil", "HigherLevel"=FALSE, "prev_pnt"=0, "last_pnt"=0} ("AverageAction"), "HigherLevel"=w413, "prev_pnt"=w414, "Level"=typedef_Level."L7_PAQ_1day", "last_pnt"=w415) -> (w420:T2)
              }
            }
          }
          frame "L7_PAQ_1day" {
            w450 = 86400.0  # +1day
            w454 = 7  # L7_1day
            w456 = 6  # L6_2hr
            # "week sat/sun passing"
            n190 = Unbundle By Name(w462) -> ("TagIndex"=w466:i32[])
            n191 = Unbundle By Name(w467) -> ("prev_pnt"=w464:i32, "last_pnt"=w463:i32)
            n192 = Unbundle By Name(w462) -> ("Time"=w451:dbl)
            n193 = Add(x=w450, y=w451) -> (x+y=w449:dbl)
            n194 = Index Array(array=w471, index #1=w454, index #2=w456) -> (element #1=w458:refnum<data-value>, element #2=w457:refnum<data-value>)
            n195 = Bundle By Name(cluster=T4 {"TAGs"=[], "prev_pnt"=0, "last_pnt"=0} ("ChunkDefinition"), "TAGs"=w466, "prev_pnt"=w464, "last_pnt"=w463) -> (w459:T4)
            n196 = To Time Stamp(1:w449) -> (0:w453:timestamp)
            n197 = Format Into String(format string="%<%W-%y>T", w453) -> (resulting string=w446:string)  [unwired: 2 in, 1 out]
            n198 = in-place {
              in-place-border: w462 -> [w506]
              in-place-border: [w501] -> w455
              in-place-border: w459 -> [w499]
              in-place-border: [w497] -> w448
              n199 = in-place-dvr #36(w457) -> (w509:refnum<class "PAQ-memory.lvclass">)  [unwired: 1 out]
              n200 = in-place-match #37(w461) -> (w508:errorcluster)
              n201 = call "PAQmem_ReadAverage.vi"("error in (no error)"=w508, "ChunkDefinition"=w499, "PAQ-memory in"=w509) -> ("error out"=w507:errorcluster, "Results"=w510:T7, "PAQ-memory out"=w500:refnum<class "PAQ-memory.lvclass">)  [unwired: 6 in]
              n202 = Unbundle By Name(w510) -> ("data"=w505:dbl[], "max"=w504:dbl[], "min"=w503:dbl[], "status"=w502:u32[], "Time"=w498:dbl)
              n203 = Not Equal To 0?(x=w498) -> (x != 0?=w497:bool)
              n204 = Bundle By Name(cluster=w506, "data"=w505, "max"=w504, "min"=w503, "status"=w502, "Time"=w498) -> (w501:T3)
              n205 = in-place-dvr #36(w500) -> ()  [unwired: 2 out]
              n206 = in-place-match #37(w507) -> (w460:errorcluster)
            }
            n207 = feedback #38() -> (w447:string)  [unwired: 1 in]
            n208 = feedback-in #38(w446) -> ()
            n209 = Not Equal?(x=w446, y=w447) -> (x != y?=w445:bool)
            n210 = case "Averaging data valid?" shown="True" w448 {
              selector: w448 -> [w476 _]
              tunnel: [w475 w488] -> w472
              tunnel: [w474 w486] -> w470
              tunnel: w469 -> [w473 w480]
              tunnel: [w473 w480] -> w468
              tunnel: w460 -> [w475 w485]
              tunnel: w458 -> [_ w484]
              tunnel: w455 -> [_ w483]
              tunnel: w445 -> [_ w479]
              frame False {
                n211 = Bundle By Name(cluster=T2 {"Level"=enum."L0_PAQ_10mil", "HigherLevel"=FALSE, "prev_pnt"=0, "last_pnt"=0} ("AverageAction"), "HigherLevel"=w476) -> (w474:T2)
              }
              frame True {
                n212 = in-place {
                  in-place-border: w483 -> [w491]
                  in-place-border: [w494] -> w481
                  in-place-border: w479 -> [w490]
                  in-place-border: [w489] -> w478
                  n213 = in-place-dvr #39(w484) -> (w493:refnum<class "PAQ-memory.lvclass">)  [unwired: 1 out]
                  n214 = in-place-match #40(w485) -> (w492:errorcluster)
                  n215 = call "PAQmem_WriteOne.vi"("Carry"=w490, "error in (no error)"=w492, "StoreDatagram"=w491, "PAQ-memory in"=w493) -> ("error out"=w495:errorcluster, "Last"=w494:i32, "Prev"=w489:i32, "PAQ-memory out"=w496:refnum<class "PAQ-memory.lvclass">)  [unwired: 4 in]
                  n216 = in-place-dvr #39(w496) -> ()  [unwired: 2 out]
                  n217 = in-place-match #40(w495) -> (w488:errorcluster)
                }
                n218 = Bundle By Name(cluster=T2 {"Level"=enum."L0_PAQ_10mil", "HigherLevel"=FALSE, "prev_pnt"=0, "last_pnt"=0} ("AverageAction"), "HigherLevel"=w479, "prev_pnt"=w478, "Level"=typedef_Level."L8_PAQ_1wk", "last_pnt"=w481) -> (w486:T2)
              }
            }
          }
          frame "L8_PAQ_1wk" {
            w512 = 8  # L8_1wk
            w514 = 7  # L7_1day
            n219 = Unbundle By Name(w520) -> ("TagIndex"=w524:i32[])
            n220 = Unbundle By Name(w525) -> ("prev_pnt"=w522:i32, "last_pnt"=w521:i32)
            n221 = Index Array(array=w529, index #1=w512, index #2=w514) -> (element #1=w516:refnum<data-value>, element #2=w515:refnum<data-value>)
            n222 = Bundle By Name(cluster=T4 {"TAGs"=[], "prev_pnt"=0, "last_pnt"=0} ("ChunkDefinition"), "TAGs"=w524, "prev_pnt"=w522, "last_pnt"=w521) -> (w517:T4)
            n223 = in-place {
              in-place-border: w520 -> [w559]
              in-place-border: [w554] -> w513
              in-place-border: w517 -> [w552]
              in-place-border: [w550] -> w511
              n224 = in-place-dvr #41(w515) -> (w562:refnum<class "PAQ-memory.lvclass">)  [unwired: 1 out]
              n225 = in-place-match #42(w519) -> (w561:errorcluster)
              n226 = call "PAQmem_ReadAverage.vi"("error in (no error)"=w561, "ChunkDefinition"=w552, "PAQ-memory in"=w562) -> ("error out"=w560:errorcluster, "Results"=w563:T7, "PAQ-memory out"=w553:refnum<class "PAQ-memory.lvclass">)  [unwired: 6 in]
              n227 = Unbundle By Name(w563) -> ("data"=w558:dbl[], "max"=w557:dbl[], "min"=w556:dbl[], "status"=w555:u32[], "Time"=w551:dbl)
              n228 = Not Equal To 0?(x=w551) -> (x != 0?=w550:bool)
              n229 = Bundle By Name(cluster=w559, "data"=w558, "max"=w557, "min"=w556, "status"=w555, "Time"=w551) -> (w554:T3)
              n230 = in-place-dvr #41(w553) -> ()  [unwired: 2 out]
              n231 = in-place-match #42(w560) -> (w518:errorcluster)
            }
            n232 = case "Averaging data valid?" shown="True" w511 {
              selector: w511 -> [w531 _]
              tunnel: [w534 w543] -> w530
              tunnel: [w532 w541] -> w528
              tunnel: w527 -> [w535 w537]
              tunnel: [w535 w537] -> w526
              tunnel: w518 -> [w534 w540]
              tunnel: w516 -> [_ w539]
              tunnel: w513 -> [_ w538]
              frame False {
                n233 = Bundle By Name(cluster=T2 {"Level"=enum."L0_PAQ_10mil", "HigherLevel"=FALSE, "prev_pnt"=0, "last_pnt"=0} ("AverageAction"), "HigherLevel"=w531) -> (w532:T2)
              }
              frame True {
                w536 = FALSE
                n234 = in-place {
                  in-place-border: w538 -> [w545]
                  in-place-border: w536 -> [w544]
                  n235 = in-place-dvr #43(w539) -> (w547:refnum<class "PAQ-memory.lvclass">)  [unwired: 1 out]
                  n236 = in-place-match #44(w540) -> (w546:errorcluster)
                  n237 = call "PAQmem_WriteOne.vi"("Carry"=w544, "error in (no error)"=w546, "StoreDatagram"=w545, "PAQ-memory in"=w547) -> ("error out"=w548:errorcluster, "PAQ-memory out"=w549:refnum<class "PAQ-memory.lvclass">)  [unwired: 4 in, 2 out]
                  n238 = in-place-dvr #43(w549) -> ()  [unwired: 2 out]
                  n239 = in-place-match #44(w548) -> (w543:errorcluster)
                }
                n240 = Bundle By Name(cluster=T2 {"Level"=enum."L0_PAQ_10mil", "HigherLevel"=FALSE, "prev_pnt"=0, "last_pnt"=0} ("AverageAction"), "HigherLevel"=w536) -> (w541:T2)
              }
            }
          }
          frame "L0_PAQ_100mil" {
            w568 = 0  # L0_100mil
            # "T - 0.5 sec\nup to\nT + 0.5 sec"
            n241 = Unbundle By Name(w570) -> ("Time"=w575:dbl)
            n242 = Subtract(x=w575, y=0.5) -> (x-y=w573:dbl)
            n243 = Quotient & Remainder(x=w573, y=1.0) -> (floor(x/y)=w572:dbl)  [unwired: 1 out]
            n244 = Index Array(array=w580, index=w568) -> (element=w579:refnum<data-value>)
            n245 = feedback #45() -> (w571:dbl)  [unwired: 1 in]
            n246 = feedback-in #45(w572) -> ()
            n247 = Not Equal?(x=w572, y=w571) -> (x != y?=w566:bool)
            n248 = in-place {
              in-place-border: w570 -> [w588]
              in-place-border: [w585] -> w567
              in-place-border: w566 -> [w584]
              in-place-border: [w583] -> w565
              n249 = in-place-dvr #46(w579) -> (w590:refnum<class "PAQ-memory.lvclass">)  [unwired: 1 out]
              n250 = in-place-match #47(w582) -> (w587:errorcluster)
              n251 = call "PAQmem_WriteOne.vi"("Carry"=w584, "error in (no error)"=w587, "StoreDatagram"=w588, "PAQ-memory in"=w590) -> ("error out"=w586:errorcluster, "Last"=w585:i32, "Prev"=w583:i32, "PAQ-memory out"=w589:refnum<class "PAQ-memory.lvclass">)  [unwired: 4 in]
              n252 = in-place-dvr #46(w589) -> ()  [unwired: 2 out]
              n253 = in-place-match #47(w586) -> (w581:errorcluster)
            }
            n254 = Bundle By Name(cluster=T2 {"Level"=enum."L0_PAQ_10mil", "HigherLevel"=FALSE, "prev_pnt"=0, "last_pnt"=0} ("AverageAction"), "HigherLevel"=w566, "prev_pnt"=w565, "last_pnt"=w567, "Level"=typedef_Level."L1_PAQ_1sec") -> (w577:T2)
          }
          frame "L1_PAQ_1sec" {
            w595 = 1  # L1_1sec
            w597 = 0  # L0_100mil
            # "T - 5 sec\nup to\nT + 5 sec"
            n255 = Unbundle By Name(w603) -> ("Time"=w611:dbl)
            n256 = Unbundle By Name(w603) -> ("TagIndex"=w607:i32[])
            n257 = Unbundle By Name(w608) -> ("prev_pnt"=w605:i32, "last_pnt"=w604:i32)
            n258 = Index Array(array=w616, index #1=w595, index #2=w597) -> (element #1=w599:refnum<data-value>, element #2=w598:refnum<data-value>)
            n259 = Subtract(x=w611, y=5.0) -> (x-y=w609:dbl)
            n260 = Bundle By Name(cluster=T4 {"TAGs"=[], "prev_pnt"=0, "last_pnt"=0} ("ChunkDefinition"), "TAGs"=w607, "prev_pnt"=w605, "last_pnt"=w604) -> (w600:T4)
            n261 = Quotient & Remainder(x=w609, y=10.0) -> (floor(x/y)=w592:dbl)  [unwired: 1 out]
            n262 = in-place {
              in-place-border: w603 -> [w651]
              in-place-border: [w646] -> w596
              in-place-border: w600 -> [w644]
              in-place-border: [w642] -> w594
              n263 = in-place-dvr #48(w598) -> (w654:refnum<class "PAQ-memory.lvclass">)  [unwired: 1 out]
              n264 = in-place-match #49(w602) -> (w653:errorcluster)
              n265 = call "PAQmem_ReadAverage.vi"("error in (no error)"=w653, "ChunkDefinition"=w644, "PAQ-memory in"=w654) -> ("error out"=w652:errorcluster, "Results"=w655:T7, "PAQ-memory out"=w645:refnum<class "PAQ-memory.lvclass">)  [unwired: 6 in]
              n266 = Unbundle By Name(w655) -> ("data"=w650:dbl[], "max"=w649:dbl[], "min"=w648:dbl[], "status"=w647:u32[], "Time"=w643:dbl)
              n267 = Not Equal To 0?(x=w643) -> (x != 0?=w642:bool)
              n268 = Bundle By Name(cluster=w651, "data"=w650, "max"=w649, "min"=w648, "status"=w647, "Time"=w643) -> (w646:T3)
              n269 = in-place-dvr #48(w645) -> ()  [unwired: 2 out]
              n270 = in-place-match #49(w652) -> (w601:errorcluster)
            }
            n271 = feedback #50() -> (w593:dbl)  [unwired: 1 in]
            n272 = feedback-in #50(w592) -> ()
            n273 = Not Equal?(x=w592, y=w593) -> (x != y?=w591:bool)
            n274 = case "Averaging data valid?" shown="True" w594 {
              selector: w594 -> [w619 _]
              tunnel: [w621 w633] -> w617
              tunnel: [w618 w631] -> w615
              tunnel: w614 -> [w622 w623]
              tunnel: [w622 w623] -> w613
              tunnel: w601 -> [w621 w630]
              tunnel: w599 -> [_ w629]
              tunnel: w596 -> [_ w628]
              tunnel: w591 -> [_ w625]
              frame False {
                n275 = Bundle By Name(cluster=T2 {"Level"=enum."L0_PAQ_10mil", "HigherLevel"=FALSE, "prev_pnt"=0, "last_pnt"=0} ("AverageAction"), "HigherLevel"=w619) -> (w618:T2)
              }
              frame True {
                n276 = in-place {
                  in-place-border: w628 -> [w636]
                  in-place-border: [w639] -> w626
                  in-place-border: w625 -> [w635]
                  in-place-border: [w634] -> w624
                  n277 = in-place-dvr #51(w629) -> (w638:refnum<class "PAQ-memory.lvclass">)  [unwired: 1 out]
                  n278 = in-place-match #52(w630) -> (w637:errorcluster)
                  n279 = call "PAQmem_WriteOne.vi"("Carry"=w635, "error in (no error)"=w637, "StoreDatagram"=w636, "PAQ-memory in"=w638) -> ("error out"=w640:errorcluster, "Last"=w639:i32, "Prev"=w634:i32, "PAQ-memory out"=w641:refnum<class "PAQ-memory.lvclass">)  [unwired: 4 in]
                  n280 = in-place-dvr #51(w641) -> ()  [unwired: 2 out]
                  n281 = in-place-match #52(w640) -> (w633:errorcluster)
                }
                n282 = Bundle By Name(cluster=T2 {"Level"=enum."L0_PAQ_10mil", "HigherLevel"=FALSE, "prev_pnt"=0, "last_pnt"=0} ("AverageAction"), "HigherLevel"=w625, "prev_pnt"=w624, "Level"=typedef_Level."L2_PAQ_10sec", "last_pnt"=w626) -> (w631:T2)
              }
            }
          }
          frame "L2_PAQ_10sec" {
            w660 = 2  # L2_10sec
            w662 = 1  # L1_1sec
            # "T - 30 sec\nup to\nT + 30 sec"
            n283 = Unbundle By Name(w668) -> ("Time"=w676:dbl)
            n284 = Unbundle By Name(w668) -> ("TagIndex"=w672:i32[])
            n285 = Unbundle By Name(w673) -> ("prev_pnt"=w670:i32, "last_pnt"=w669:i32)
            n286 = Index Array(array=w681, index #1=w660, index #2=w662) -> (element #1=w664:refnum<data-value>, element #2=w663:refnum<data-value>)
            n287 = Subtract(x=w676, y=30.0) -> (x-y=w674:dbl)
            n288 = Bundle By Name(cluster=T4 {"TAGs"=[], "prev_pnt"=0, "last_pnt"=0} ("ChunkDefinition"), "TAGs"=w672, "prev_pnt"=w670, "last_pnt"=w669) -> (w665:T4)
            n289 = Quotient & Remainder(x=w674, y=60.0) -> (floor(x/y)=w657:dbl)  [unwired: 1 out]
            n290 = in-place {
              in-place-border: w668 -> [w715]
              in-place-border: [w710] -> w661
              in-place-border: w665 -> [w708]
              in-place-border: [w706] -> w659
              n291 = in-place-dvr #53(w663) -> (w718:refnum<class "PAQ-memory.lvclass">)  [unwired: 1 out]
              n292 = in-place-match #54(w667) -> (w717:errorcluster)
              n293 = call "PAQmem_ReadAverage.vi"("error in (no error)"=w717, "ChunkDefinition"=w708, "PAQ-memory in"=w718) -> ("error out"=w716:errorcluster, "Results"=w719:T7, "PAQ-memory out"=w709:refnum<class "PAQ-memory.lvclass">)  [unwired: 6 in]
              n294 = Unbundle By Name(w719) -> ("data"=w714:dbl[], "max"=w713:dbl[], "min"=w712:dbl[], "status"=w711:u32[], "Time"=w707:dbl)
              n295 = Not Equal To 0?(x=w707) -> (x != 0?=w706:bool)
              n296 = Bundle By Name(cluster=w715, "data"=w714, "max"=w713, "min"=w712, "status"=w711, "Time"=w707) -> (w710:T3)
              n297 = in-place-dvr #53(w709) -> ()  [unwired: 2 out]
              n298 = in-place-match #54(w716) -> (w666:errorcluster)
            }
            n299 = feedback #55() -> (w658:dbl)  [unwired: 1 in]
            n300 = feedback-in #55(w657) -> ()
            n301 = Not Equal?(x=w657, y=w658) -> (x != y?=w656:bool)
            n302 = case "Averaging data valid?" shown="True" w659 {
              selector: w659 -> [w683 _]
              tunnel: [w686 w698] -> w682
              tunnel: [w684 w696] -> w680
              tunnel: w679 -> [w687 w689]
              tunnel: [w687 w689] -> w678
              tunnel: w666 -> [w686 w695]
              tunnel: w664 -> [_ w694]
              tunnel: w661 -> [_ w693]
              tunnel: w656 -> [_ w690]
              frame False {
                n303 = Bundle By Name(cluster=T2 {"Level"=enum."L0_PAQ_10mil", "HigherLevel"=FALSE, "prev_pnt"=0, "last_pnt"=0} ("AverageAction"), "HigherLevel"=w683) -> (w684:T2)
              }
              frame True {
                n304 = in-place {
                  in-place-border: w693 -> [w700]
                  in-place-border: [w703] -> w691
                  in-place-border: [w699] -> w688
                  n305 = in-place-dvr #56(w694) -> (w702:refnum<class "PAQ-memory.lvclass">)  [unwired: 1 out]
                  n306 = in-place-match #57(w695) -> (w701:errorcluster)
                  n307 = call "PAQmem_WriteOne.vi"("error in (no error)"=w701, "StoreDatagram"=w700, "PAQ-memory in"=w702) -> ("error out"=w704:errorcluster, "Last"=w703:i32, "Prev"=w699:i32, "PAQ-memory out"=w705:refnum<class "PAQ-memory.lvclass">)  [unwired: 5 in]
                  n308 = in-place-dvr #56(w705) -> ()  [unwired: 2 out]
                  n309 = in-place-match #57(w704) -> (w698:errorcluster)
                }
                n310 = Bundle By Name(cluster=T2 {"Level"=enum."L0_PAQ_10mil", "HigherLevel"=FALSE, "prev_pnt"=0, "last_pnt"=0} ("AverageAction"), "HigherLevel"=w690, "prev_pnt"=w688, "Level"=typedef_Level."L3_PAQ_1min", "last_pnt"=w691) -> (w696:T2)
              }
            }
          }
          frame "L3_PAQ_1min" {
            w724 = 3  # L3_1min
            w726 = 2  # L2_10sec
            # "T - 5 min\nup to\nT + 5 min"
            n311 = Unbundle By Name(w732) -> ("Time"=w740:dbl)
            n312 = Unbundle By Name(w732) -> ("TagIndex"=w736:i32[])
            n313 = Unbundle By Name(w737) -> ("prev_pnt"=w734:i32, "last_pnt"=w733:i32)
            n314 = Index Array(array=w745, index #1=w724, index #2=w726) -> (element #1=w728:refnum<data-value>, element #2=w727:refnum<data-value>)
            n315 = Subtract(x=w740, y=150.0) -> (x-y=w738:dbl)
            n316 = Bundle By Name(cluster=T4 {"TAGs"=[], "prev_pnt"=0, "last_pnt"=0} ("ChunkDefinition"), "TAGs"=w736, "prev_pnt"=w734, "last_pnt"=w733) -> (w729:T4)
            n317 = Quotient & Remainder(x=w738, y=300.0) -> (floor(x/y)=w721:dbl)  [unwired: 1 out]
            n318 = in-place {
              in-place-border: w732 -> [w780]
              in-place-border: [w775] -> w725
              in-place-border: w729 -> [w773]
              in-place-border: [w771] -> w723
              n319 = in-place-dvr #58(w727) -> (w783:refnum<class "PAQ-memory.lvclass">)  [unwired: 1 out]
              n320 = in-place-match #59(w731) -> (w782:errorcluster)
              n321 = call "PAQmem_ReadAverage.vi"("error in (no error)"=w782, "ChunkDefinition"=w773, "PAQ-memory in"=w783) -> ("error out"=w781:errorcluster, "Results"=w784:T7, "PAQ-memory out"=w774:refnum<class "PAQ-memory.lvclass">)  [unwired: 6 in]
              n322 = Unbundle By Name(w784) -> ("data"=w779:dbl[], "max"=w778:dbl[], "min"=w777:dbl[], "status"=w776:u32[], "Time"=w772:dbl)
              n323 = Not Equal To 0?(x=w772) -> (x != 0?=w771:bool)
              n324 = Bundle By Name(cluster=w780, "data"=w779, "max"=w778, "min"=w777, "status"=w776, "Time"=w772) -> (w775:T3)
              n325 = in-place-dvr #58(w774) -> ()  [unwired: 2 out]
              n326 = in-place-match #59(w781) -> (w730:errorcluster)
            }
            n327 = feedback #60() -> (w722:dbl)  [unwired: 1 in]
            n328 = feedback-in #60(w721) -> ()
            n329 = Not Equal?(x=w721, y=w722) -> (x != y?=w720:bool)
            n330 = case "Averaged data valid?" shown="True" w723 {
              selector: w723 -> [w748 _]
              tunnel: [w750 w762] -> w746
              tunnel: [w747 w760] -> w744
              tunnel: w743 -> [w751 w754]
              tunnel: [w751 w754] -> w742
              tunnel: w730 -> [w750 w759]
              tunnel: w728 -> [_ w758]
              tunnel: w725 -> [_ w757]
              tunnel: w720 -> [_ w753]
              frame False {
                n331 = Bundle By Name(cluster=T2 {"Level"=enum."L0_PAQ_10mil", "HigherLevel"=FALSE, "prev_pnt"=0, "last_pnt"=0} ("AverageAction"), "HigherLevel"=w748) -> (w747:T2)
              }
              frame True {
                n332 = in-place {
                  in-place-border: w757 -> [w765]
                  in-place-border: [w768] -> w755
                  in-place-border: w753 -> [w764]
                  in-place-border: [w763] -> w752
                  n333 = in-place-dvr #61(w758) -> (w767:refnum<class "PAQ-memory.lvclass">)  [unwired: 1 out]
                  n334 = in-place-match #62(w759) -> (w766:errorcluster)
                  n335 = call "PAQmem_WriteOne.vi"("Carry"=w764, "error in (no error)"=w766, "StoreDatagram"=w765, "PAQ-memory in"=w767) -> ("error out"=w769:errorcluster, "Last"=w768:i32, "Prev"=w763:i32, "PAQ-memory out"=w770:refnum<class "PAQ-memory.lvclass">)  [unwired: 4 in]
                  n336 = in-place-dvr #61(w770) -> ()  [unwired: 2 out]
                  n337 = in-place-match #62(w769) -> (w762:errorcluster)
                }
                n338 = Bundle By Name(cluster=T2 {"Level"=enum."L0_PAQ_10mil", "HigherLevel"=FALSE, "prev_pnt"=0, "last_pnt"=0} ("AverageAction"), "HigherLevel"=w753, "prev_pnt"=w752, "Level"=typedef_Level."L4_PAQ_10min", "last_pnt"=w755) -> (w760:T2)
              }
            }
          }
          frame "L4_PAQ_10min" {
            w789 = 4  # L4_10min
            w791 = 3  # L3_1min
            # "T - 1 hr\nup to\nT + 1 hr"
            n339 = Unbundle By Name(w797) -> ("Time"=w805:dbl)
            n340 = Unbundle By Name(w797) -> ("TagIndex"=w801:i32[])
            n341 = Unbundle By Name(w802) -> ("prev_pnt"=w799:i32, "last_pnt"=w798:i32)
            n342 = Index Array(array=w810, index #1=w789, index #2=w791) -> (element #1=w793:refnum<data-value>, element #2=w792:refnum<data-value>)
            n343 = Subtract(x=w805, y=1800.0) -> (x-y=w803:dbl)
            n344 = Bundle By Name(cluster=T4 {"TAGs"=[], "prev_pnt"=0, "last_pnt"=0} ("ChunkDefinition"), "TAGs"=w801, "prev_pnt"=w799, "last_pnt"=w798) -> (w794:T4)
            n345 = Quotient & Remainder(x=w803, y=3600.0) -> (floor(x/y)=w786:dbl)  [unwired: 1 out]
            n346 = in-place {
              in-place-border: w797 -> [w845]
              in-place-border: [w840] -> w790
              in-place-border: w794 -> [w838]
              in-place-border: [w836] -> w788
              n347 = in-place-dvr #63(w792) -> (w848:refnum<class "PAQ-memory.lvclass">)  [unwired: 1 out]
              n348 = in-place-match #64(w796) -> (w847:errorcluster)
              n349 = call "PAQmem_ReadAverage.vi"("error in (no error)"=w847, "ChunkDefinition"=w838, "PAQ-memory in"=w848) -> ("error out"=w846:errorcluster, "Results"=w849:T7, "PAQ-memory out"=w839:refnum<class "PAQ-memory.lvclass">)  [unwired: 6 in]
              n350 = Unbundle By Name(w849) -> ("data"=w844:dbl[], "max"=w843:dbl[], "min"=w842:dbl[], "status"=w841:u32[], "Time"=w837:dbl)
              n351 = Not Equal To 0?(x=w837) -> (x != 0?=w836:bool)
              n352 = Bundle By Name(cluster=w845, "data"=w844, "max"=w843, "min"=w842, "status"=w841, "Time"=w837) -> (w840:T3)
              n353 = in-place-dvr #63(w839) -> ()  [unwired: 2 out]
              n354 = in-place-match #64(w846) -> (w795:errorcluster)
            }
            n355 = feedback #65() -> (w787:dbl)  [unwired: 1 in]
            n356 = feedback-in #65(w786) -> ()
            n357 = Not Equal?(x=w786, y=w787) -> (x != y?=w785:bool)
            n358 = case "Averaged data valid?" shown="True" w788 {
              selector: w788 -> [w814 _]
              tunnel: [w813 w827] -> w811
              tunnel: [w815 w825] -> w809
              tunnel: w808 -> [w812 w819]
              tunnel: [w812 w819] -> w807
              tunnel: w795 -> [w813 w824]
              tunnel: w793 -> [_ w823]
              tunnel: w790 -> [_ w822]
              tunnel: w785 -> [_ w818]
              frame False {
                n359 = Bundle By Name(cluster=T2 {"Level"=enum."L0_PAQ_10mil", "HigherLevel"=FALSE, "prev_pnt"=0, "last_pnt"=0} ("AverageAction"), "HigherLevel"=w814) -> (w815:T2)
              }
              frame True {
                n360 = in-place {
                  in-place-border: w822 -> [w830]
                  in-place-border: [w833] -> w820
                  in-place-border: w818 -> [w829]
                  in-place-border: [w828] -> w817
                  n361 = in-place-dvr #66(w823) -> (w832:refnum<class "PAQ-memory.lvclass">)  [unwired: 1 out]
                  n362 = in-place-match #67(w824) -> (w831:errorcluster)
                  n363 = call "PAQmem_WriteOne.vi"("Carry"=w829, "error in (no error)"=w831, "StoreDatagram"=w830, "PAQ-memory in"=w832) -> ("error out"=w834:errorcluster, "Last"=w833:i32, "Prev"=w828:i32, "PAQ-memory out"=w835:refnum<class "PAQ-memory.lvclass">)  [unwired: 4 in]
                  n364 = in-place-dvr #66(w835) -> ()  [unwired: 2 out]
                  n365 = in-place-match #67(w834) -> (w827:errorcluster)
                }
                n366 = Bundle By Name(cluster=T2 {"Level"=enum."L0_PAQ_10mil", "HigherLevel"=FALSE, "prev_pnt"=0, "last_pnt"=0} ("AverageAction"), "HigherLevel"=w818, "prev_pnt"=w817, "Level"=typedef_Level."L5_PAQ_2hr", "last_pnt"=w820) -> (w825:T2)
              }
            }
          }
          frame "L5_PAQ_2hr" {
            w857 = 5  # L5_2hr
            w859 = 4  # L4_10min
            # "check day passing"
            n367 = Unbundle By Name(w865) -> ("TagIndex"=w869:i32[])
            n368 = Unbundle By Name(w870) -> ("prev_pnt"=w867:i32, "last_pnt"=w866:i32)
            n369 = Unbundle By Name(w865) -> ("Time"=w856:dbl)
            n370 = To Time Stamp(1:w856) -> (0:w855:timestamp)
            n371 = Index Array(array=w874, index #1=w857, index #2=w859) -> (element #1=w861:refnum<data-value>, element #2=w860:refnum<data-value>)
            n372 = Format Into String(format string="%<%d-%m-%y>T", w855) -> (resulting string=w851:string)  [unwired: 2 in, 1 out]
            n373 = Bundle By Name(cluster=T4 {"TAGs"=[], "prev_pnt"=0, "last_pnt"=0} ("ChunkDefinition"), "TAGs"=w869, "prev_pnt"=w867, "last_pnt"=w866) -> (w862:T4)
            n374 = in-place {
              in-place-border: w865 -> [w909]
              in-place-border: [w904] -> w858
              in-place-border: w862 -> [w902]
              in-place-border: [w900] -> w853
              n375 = in-place-dvr #68(w860) -> (w912:refnum<class "PAQ-memory.lvclass">)  [unwired: 1 out]
              n376 = in-place-match #69(w864) -> (w911:errorcluster)
              n377 = call "PAQmem_ReadAverage.vi"("error in (no error)"=w911, "ChunkDefinition"=w902, "PAQ-memory in"=w912) -> ("error out"=w910:errorcluster, "Results"=w913:T7, "PAQ-memory out"=w903:refnum<class "PAQ-memory.lvclass">)  [unwired: 6 in]
              n378 = Unbundle By Name(w913) -> ("data"=w908:dbl[], "max"=w907:dbl[], "min"=w906:dbl[], "status"=w905:u32[], "Time"=w901:dbl)
              n379 = Not Equal To 0?(x=w901) -> (x != 0?=w900:bool)
              n380 = Bundle By Name(cluster=w909, "data"=w908, "max"=w907, "min"=w906, "status"=w905, "Time"=w901) -> (w904:T3)
              n381 = in-place-dvr #68(w903) -> ()  [unwired: 2 out]
              n382 = in-place-match #69(w910) -> (w863:errorcluster)
            }
            n383 = feedback #70() -> (w852:string)  [unwired: 1 in]
            n384 = feedback-in #70(w851) -> ()
            n385 = Not Equal?(x=w851, y=w852) -> (x != y?=w850:bool)
            n386 = case "Averaged data valid?" shown="True" w853 {
              selector: w853 -> [w877 _]
              tunnel: [w879 w891] -> w875
              tunnel: [w876 w889] -> w873
              tunnel: w872 -> [w880 w881]
              tunnel: [w880 w881] -> w871
              tunnel: w863 -> [w879 w888]
              tunnel: w861 -> [_ w887]
              tunnel: w858 -> [_ w886]
              tunnel: w850 -> [_ w883]
              frame False {
                n387 = Bundle By Name(cluster=T2 {"Level"=enum."L0_PAQ_10mil", "HigherLevel"=FALSE, "prev_pnt"=0, "last_pnt"=0} ("AverageAction"), "HigherLevel"=w877) -> (w876:T2)
              }
              frame True {
                n388 = in-place {
                  in-place-border: w886 -> [w894]
                  in-place-border: [w897] -> w884
                  in-place-border: w883 -> [w893]
                  in-place-border: [w892] -> w882
                  n389 = in-place-dvr #71(w887) -> (w896:refnum<class "PAQ-memory.lvclass">)  [unwired: 1 out]
                  n390 = in-place-match #72(w888) -> (w895:errorcluster)
                  n391 = call "PAQmem_WriteOne.vi"("Carry"=w893, "error in (no error)"=w895, "StoreDatagram"=w894, "PAQ-memory in"=w896) -> ("error out"=w898:errorcluster, "Last"=w897:i32, "Prev"=w892:i32, "PAQ-memory out"=w899:refnum<class "PAQ-memory.lvclass">)  [unwired: 4 in]
                  n392 = in-place-dvr #71(w899) -> ()  [unwired: 2 out]
                  n393 = in-place-match #72(w898) -> (w891:errorcluster)
                }
                n394 = Bundle By Name(cluster=T2 {"Level"=enum."L0_PAQ_10mil", "HigherLevel"=FALSE, "prev_pnt"=0, "last_pnt"=0} ("AverageAction"), "HigherLevel"=w883, "prev_pnt"=w882, "Level"=typedef_Level."L6_PAQ_1day", "last_pnt"=w884) -> (w889:T2)
              }
            }
          }
          frame "L6_PAQ_1day" {
            w919 = 86400.0  # +1day
            w923 = 6  # L6_1day
            w925 = 5  # L5_2hr
            # "week sat/sun passing"
            n395 = Unbundle By Name(w931) -> ("TagIndex"=w935:i32[])
            n396 = Unbundle By Name(w936) -> ("prev_pnt"=w933:i32, "last_pnt"=w932:i32)
            n397 = Unbundle By Name(w931) -> ("Time"=w920:dbl)
            n398 = Add(x=w919, y=w920) -> (x+y=w918:dbl)
            n399 = Index Array(array=w940, index #1=w923, index #2=w925) -> (element #1=w927:refnum<data-value>, element #2=w926:refnum<data-value>)
            n400 = Bundle By Name(cluster=T4 {"TAGs"=[], "prev_pnt"=0, "last_pnt"=0} ("ChunkDefinition"), "TAGs"=w935, "prev_pnt"=w933, "last_pnt"=w932) -> (w928:T4)
            n401 = To Time Stamp(1:w918) -> (0:w922:timestamp)
            n402 = Format Into String(format string="%<%W-%y>T", w922) -> (resulting string=w915:string)  [unwired: 2 in, 1 out]
            n403 = in-place {
              in-place-border: w931 -> [w975]
              in-place-border: [w970] -> w924
              in-place-border: w928 -> [w968]
              in-place-border: [w966] -> w917
              n404 = in-place-dvr #73(w926) -> (w978:refnum<class "PAQ-memory.lvclass">)  [unwired: 1 out]
              n405 = in-place-match #74(w930) -> (w977:errorcluster)
              n406 = call "PAQmem_ReadAverage.vi"("error in (no error)"=w977, "ChunkDefinition"=w968, "PAQ-memory in"=w978) -> ("error out"=w976:errorcluster, "Results"=w979:T7, "PAQ-memory out"=w969:refnum<class "PAQ-memory.lvclass">)  [unwired: 6 in]
              n407 = Unbundle By Name(w979) -> ("data"=w974:dbl[], "max"=w973:dbl[], "min"=w972:dbl[], "status"=w971:u32[], "Time"=w967:dbl)
              n408 = Not Equal To 0?(x=w967) -> (x != 0?=w966:bool)
              n409 = Bundle By Name(cluster=w975, "data"=w974, "max"=w973, "min"=w972, "status"=w971, "Time"=w967) -> (w970:T3)
              n410 = in-place-dvr #73(w969) -> ()  [unwired: 2 out]
              n411 = in-place-match #74(w976) -> (w929:errorcluster)
            }
            n412 = feedback #75() -> (w916:string)  [unwired: 1 in]
            n413 = feedback-in #75(w915) -> ()
            n414 = Not Equal?(x=w915, y=w916) -> (x != y?=w914:bool)
            n415 = case "Averaged data valid?" shown="True" w917 {
              selector: w917 -> [w945 _]
              tunnel: [w942 w957] -> w941
              tunnel: [w944 w955] -> w939
              tunnel: w938 -> [w943 w949]
              tunnel: [w943 w949] -> w937
              tunnel: w929 -> [w942 w954]
              tunnel: w927 -> [_ w953]
              tunnel: w924 -> [_ w952]
              tunnel: w914 -> [_ w947]
              frame False {
                n416 = Bundle By Name(cluster=T2 {"Level"=enum."L0_PAQ_10mil", "HigherLevel"=FALSE, "prev_pnt"=0, "last_pnt"=0} ("AverageAction"), "HigherLevel"=w945) -> (w944:T2)
              }
              frame True {
                n417 = in-place {
                  in-place-border: w952 -> [w960]
                  in-place-border: [w963] -> w950
                  in-place-border: [w959] -> w948
                  in-place-border: w947 -> [w958]
                  n418 = in-place-dvr #76(w953) -> (w962:refnum<class "PAQ-memory.lvclass">)  [unwired: 1 out]
                  n419 = in-place-match #77(w954) -> (w961:errorcluster)
                  n420 = call "PAQmem_WriteOne.vi"("Carry"=w958, "error in (no error)"=w961, "StoreDatagram"=w960, "PAQ-memory in"=w962) -> ("error out"=w964:errorcluster, "Last"=w963:i32, "Prev"=w959:i32, "PAQ-memory out"=w965:refnum<class "PAQ-memory.lvclass">)  [unwired: 4 in]
                  n421 = in-place-dvr #76(w965) -> ()  [unwired: 2 out]
                  n422 = in-place-match #77(w964) -> (w957:errorcluster)
                }
                n423 = Bundle By Name(cluster=T2 {"Level"=enum."L0_PAQ_10mil", "HigherLevel"=FALSE, "prev_pnt"=0, "last_pnt"=0} ("AverageAction"), "HigherLevel"=w947, "prev_pnt"=w948, "Level"=typedef_Level."L7_PAQ_1wk", "last_pnt"=w950) -> (w955:T2)
              }
            }
          }
          frame "L7_PAQ_1wk" {
            w981 = 7  # L7_1wk
            w983 = 6  # L6_1day
            n424 = Unbundle By Name(w989) -> ("TagIndex"=w993:i32[])
            n425 = Unbundle By Name(w994) -> ("prev_pnt"=w991:i32, "last_pnt"=w990:i32)
            n426 = Index Array(array=w998, index #1=w981, index #2=w983) -> (element #1=w985:refnum<data-value>, element #2=w984:refnum<data-value>)
            n427 = Bundle By Name(cluster=T4 {"TAGs"=[], "prev_pnt"=0, "last_pnt"=0} ("ChunkDefinition"), "TAGs"=w993, "prev_pnt"=w991, "last_pnt"=w990) -> (w986:T4)
            n428 = in-place {
              in-place-border: w989 -> [w1028]
              in-place-border: [w1023] -> w982
              in-place-border: w986 -> [w1021]
              in-place-border: [w1019] -> w980
              n429 = in-place-dvr #78(w984) -> (w1031:refnum<class "PAQ-memory.lvclass">)  [unwired: 1 out]
              n430 = in-place-match #79(w988) -> (w1030:errorcluster)
              n431 = call "PAQmem_ReadAverage.vi"("error in (no error)"=w1030, "ChunkDefinition"=w1021, "PAQ-memory in"=w1031) -> ("error out"=w1029:errorcluster, "Results"=w1032:T7, "PAQ-memory out"=w1022:refnum<class "PAQ-memory.lvclass">)  [unwired: 6 in]
              n432 = Unbundle By Name(w1032) -> ("data"=w1027:dbl[], "max"=w1026:dbl[], "min"=w1025:dbl[], "status"=w1024:u32[], "Time"=w1020:dbl)
              n433 = Not Equal To 0?(x=w1020) -> (x != 0?=w1019:bool)
              n434 = Bundle By Name(cluster=w1028, "data"=w1027, "max"=w1026, "min"=w1025, "status"=w1024, "Time"=w1020) -> (w1023:T3)
              n435 = in-place-dvr #78(w1022) -> ()  [unwired: 2 out]
              n436 = in-place-match #79(w1029) -> (w987:errorcluster)
            }
            n437 = case "Averaged data valid?" shown="True" w980 {
              selector: w980 -> [w1002 _]
              tunnel: [w1000 w1012] -> w999
              tunnel: [w1001 w1010] -> w997
              tunnel: w996 -> [w1004 w1005]
              tunnel: [w1004 w1005] -> w995
              tunnel: w987 -> [w1000 w1009]
              tunnel: w985 -> [_ w1008]
              tunnel: w982 -> [_ w1007]
              frame False {
                n438 = Bundle By Name(cluster=T2 {"Level"=enum."L0_PAQ_10mil", "HigherLevel"=FALSE, "prev_pnt"=0, "last_pnt"=0} ("AverageAction"), "HigherLevel"=w1002) -> (w1001:T2)
              }
              frame True {
                w1006 = FALSE
                n439 = in-place {
                  in-place-border: w1007 -> [w1014]
                  in-place-border: w1006 -> [w1013]
                  n440 = in-place-dvr #80(w1008) -> (w1016:refnum<class "PAQ-memory.lvclass">)  [unwired: 1 out]
                  n441 = in-place-match #81(w1009) -> (w1015:errorcluster)
                  n442 = call "PAQmem_WriteOne.vi"("Carry"=w1013, "error in (no error)"=w1015, "StoreDatagram"=w1014, "PAQ-memory in"=w1016) -> ("error out"=w1017:errorcluster, "PAQ-memory out"=w1018:refnum<class "PAQ-memory.lvclass">)  [unwired: 4 in, 2 out]
                  n443 = in-place-dvr #80(w1018) -> ()  [unwired: 2 out]
                  n444 = in-place-match #81(w1017) -> (w1012:errorcluster)
                }
                n445 = Bundle By Name(cluster=T2 {"Level"=enum."L0_PAQ_10mil", "HigherLevel"=FALSE, "prev_pnt"=0, "last_pnt"=0} ("AverageAction"), "HigherLevel"=w1006) -> (w1010:T2)
              }
            }
          }
          frame "L0_PAQ_1sec" {
            w1037 = 0  # L0_1sec
            # "T - 5 sec\nup to\nT + 5 sec"
            n446 = Unbundle By Name(w1039) -> ("Time"=w1044:dbl)
            n447 = Subtract(x=w1044, y=5.0) -> (x-y=w1042:dbl)
            n448 = Quotient & Remainder(x=w1042, y=10.0) -> (floor(x/y)=w1041:dbl)  [unwired: 1 out]
            n449 = Index Array(array=w1049, index=w1037) -> (element=w1048:refnum<data-value>)
            n450 = feedback #82() -> (w1040:dbl)  [unwired: 1 in]
            n451 = feedback-in #82(w1041) -> ()
            n452 = Not Equal?(x=w1041, y=w1040) -> (x != y?=w1035:bool)
            n453 = in-place {
              in-place-border: w1039 -> [w1057]
              in-place-border: [w1054] -> w1036
              in-place-border: w1035 -> [w1053]
              in-place-border: [w1052] -> w1033
              n454 = in-place-dvr #83(w1048) -> (w1059:refnum<class "PAQ-memory.lvclass">)  [unwired: 1 out]
              n455 = in-place-match #84(w1051) -> (w1056:errorcluster)
              n456 = call "PAQmem_WriteOne.vi"("Carry"=w1053, "error in (no error)"=w1056, "StoreDatagram"=w1057, "PAQ-memory in"=w1059) -> ("error out"=w1055:errorcluster, "Last"=w1054:i32, "Prev"=w1052:i32, "PAQ-memory out"=w1058:refnum<class "PAQ-memory.lvclass">)  [unwired: 4 in]
              n457 = in-place-dvr #83(w1058) -> ()  [unwired: 2 out]
              n458 = in-place-match #84(w1055) -> (w1050:errorcluster)
            }
            n459 = Bundle By Name(cluster=T2 {"Level"=enum."L0_PAQ_10mil", "HigherLevel"=FALSE, "prev_pnt"=0, "last_pnt"=0} ("AverageAction"), "HigherLevel"=w1035, "prev_pnt"=w1033, "last_pnt"=w1036, "Level"=typedef_Level."L1_PAQ_10sec") -> (w1046:T2)
          }
          frame "L1_PAQ_10sec" {
            w1064 = 1  # L1_10sec
            w1066 = 0  # L0_1sec
            # "T - 30 sec\nup to\nT + 30 sec"
            n460 = Unbundle By Name(w1072) -> ("Time"=w1080:dbl)
            n461 = Unbundle By Name(w1072) -> ("TagIndex"=w1076:i32[])
            n462 = Unbundle By Name(w1077) -> ("prev_pnt"=w1074:i32, "last_pnt"=w1073:i32)
            n463 = Index Array(array=w1085, index #1=w1064, index #2=w1066) -> (element #1=w1068:refnum<data-value>, element #2=w1067:refnum<data-value>)
            n464 = Subtract(x=w1080, y=30.0) -> (x-y=w1078:dbl)
            n465 = Bundle By Name(cluster=T4 {"TAGs"=[], "prev_pnt"=0, "last_pnt"=0} ("ChunkDefinition"), "TAGs"=w1076, "prev_pnt"=w1074, "last_pnt"=w1073) -> (w1069:T4)
            n466 = Quotient & Remainder(x=w1078, y=60.0) -> (floor(x/y)=w1061:dbl)  [unwired: 1 out]
            n467 = in-place {
              in-place-border: w1072 -> [w1120]
              in-place-border: [w1115] -> w1065
              in-place-border: w1069 -> [w1113]
              in-place-border: [w1111] -> w1063
              n468 = in-place-dvr #85(w1067) -> (w1123:refnum<class "PAQ-memory.lvclass">)  [unwired: 1 out]
              n469 = in-place-match #86(w1071) -> (w1122:errorcluster)
              n470 = call "PAQmem_ReadAverage.vi"("error in (no error)"=w1122, "ChunkDefinition"=w1113, "PAQ-memory in"=w1123) -> ("error out"=w1121:errorcluster, "Results"=w1124:T7, "PAQ-memory out"=w1114:refnum<class "PAQ-memory.lvclass">)  [unwired: 6 in]
              n471 = Unbundle By Name(w1124) -> ("data"=w1119:dbl[], "max"=w1118:dbl[], "min"=w1117:dbl[], "status"=w1116:u32[], "Time"=w1112:dbl)
              n472 = Not Equal To 0?(x=w1112) -> (x != 0?=w1111:bool)
              n473 = Bundle By Name(cluster=w1120, "data"=w1119, "max"=w1118, "min"=w1117, "status"=w1116, "Time"=w1112) -> (w1115:T3)
              n474 = in-place-dvr #85(w1114) -> ()  [unwired: 2 out]
              n475 = in-place-match #86(w1121) -> (w1070:errorcluster)
            }
            n476 = feedback #87() -> (w1062:dbl)  [unwired: 1 in]
            n477 = feedback-in #87(w1061) -> ()
            n478 = Not Equal?(x=w1061, y=w1062) -> (x != y?=w1060:bool)
            n479 = case "Averaged data valid?" shown="True" w1063 {
              selector: w1063 -> [w1090 _]
              tunnel: [w1087 w1102] -> w1086
              tunnel: [w1089 w1100] -> w1084
              tunnel: w1083 -> [w1088 w1092]
              tunnel: [w1088 w1092] -> w1082
              tunnel: w1070 -> [w1087 w1099]
              tunnel: w1068 -> [_ w1098]
              tunnel: w1065 -> [_ w1097]
              tunnel: w1060 -> [_ w1093]
              frame False {
                n480 = Bundle By Name(cluster=T2 {"Level"=enum."L0_PAQ_10mil", "HigherLevel"=FALSE, "prev_pnt"=0, "last_pnt"=0} ("AverageAction"), "HigherLevel"=w1090) -> (w1089:T2)
              }
              frame True {
                n481 = in-place {
                  in-place-border: w1097 -> [w1105]
                  in-place-border: [w1108] -> w1095
                  in-place-border: [w1104] -> w1094
                  in-place-border: w1093 -> [w1103]
                  n482 = in-place-dvr #88(w1098) -> (w1107:refnum<class "PAQ-memory.lvclass">)  [unwired: 1 out]
                  n483 = in-place-match #89(w1099) -> (w1106:errorcluster)
                  n484 = call "PAQmem_WriteOne.vi"("Carry"=w1103, "error in (no error)"=w1106, "StoreDatagram"=w1105, "PAQ-memory in"=w1107) -> ("error out"=w1109:errorcluster, "Last"=w1108:i32, "Prev"=w1104:i32, "PAQ-memory out"=w1110:refnum<class "PAQ-memory.lvclass">)  [unwired: 4 in]
                  n485 = in-place-dvr #88(w1110) -> ()  [unwired: 2 out]
                  n486 = in-place-match #89(w1109) -> (w1102:errorcluster)
                }
                n487 = Bundle By Name(cluster=T2 {"Level"=enum."L0_PAQ_10mil", "HigherLevel"=FALSE, "prev_pnt"=0, "last_pnt"=0} ("AverageAction"), "HigherLevel"=w1093, "prev_pnt"=w1094, "Level"=typedef_Level."L2_PAQ_1min", "last_pnt"=w1095) -> (w1100:T2)
              }
            }
          }
          frame "L2_PAQ_1min" {
            w1129 = 2  # L2_1min
            w1131 = 1  # L1_10sec
            # "T - 5 min\nup to\nT + 5 min"
            n488 = Unbundle By Name(w1137) -> ("Time"=w1145:dbl)
            n489 = Unbundle By Name(w1137) -> ("TagIndex"=w1141:i32[])
            n490 = Unbundle By Name(w1142) -> ("prev_pnt"=w1139:i32, "last_pnt"=w1138:i32)
            n491 = Index Array(array=w1150, index #1=w1129, index #2=w1131) -> (element #1=w1133:refnum<data-value>, element #2=w1132:refnum<data-value>)
            n492 = Subtract(x=w1145, y=150.0) -> (x-y=w1143:dbl)
            n493 = Bundle By Name(cluster=T4 {"TAGs"=[], "prev_pnt"=0, "last_pnt"=0} ("ChunkDefinition"), "TAGs"=w1141, "prev_pnt"=w1139, "last_pnt"=w1138) -> (w1134:T4)
            n494 = Quotient & Remainder(x=w1143, y=300.0) -> (floor(x/y)=w1126:dbl)  [unwired: 1 out]
            n495 = in-place {
              in-place-border: w1137 -> [w1185]
              in-place-border: [w1180] -> w1130
              in-place-border: w1134 -> [w1178]
              in-place-border: [w1176] -> w1128
              n496 = in-place-dvr #90(w1132) -> (w1188:refnum<class "PAQ-memory.lvclass">)  [unwired: 1 out]
              n497 = in-place-match #91(w1136) -> (w1187:errorcluster)
              n498 = call "PAQmem_ReadAverage.vi"("error in (no error)"=w1187, "ChunkDefinition"=w1178, "PAQ-memory in"=w1188) -> ("error out"=w1186:errorcluster, "Results"=w1189:T7, "PAQ-memory out"=w1179:refnum<class "PAQ-memory.lvclass">)  [unwired: 6 in]
              n499 = Unbundle By Name(w1189) -> ("data"=w1184:dbl[], "max"=w1183:dbl[], "min"=w1182:dbl[], "status"=w1181:u32[], "Time"=w1177:dbl)
              n500 = Not Equal To 0?(x=w1177) -> (x != 0?=w1176:bool)
              n501 = Bundle By Name(cluster=w1185, "data"=w1184, "max"=w1183, "min"=w1182, "status"=w1181, "Time"=w1177) -> (w1180:T3)
              n502 = in-place-dvr #90(w1179) -> ()  [unwired: 2 out]
              n503 = in-place-match #91(w1186) -> (w1135:errorcluster)
            }
            n504 = feedback #92() -> (w1127:dbl)  [unwired: 1 in]
            n505 = feedback-in #92(w1126) -> ()
            n506 = Not Equal?(x=w1126, y=w1127) -> (x != y?=w1125:bool)
            n507 = case "Averaged data valid?" shown="True" w1128 {
              selector: w1128 -> [w1153 _]
              tunnel: [w1155 w1167] -> w1151
              tunnel: [w1152 w1165] -> w1149
              tunnel: w1148 -> [w1156 w1159]
              tunnel: [w1156 w1159] -> w1147
              tunnel: w1135 -> [w1155 w1164]
              tunnel: w1133 -> [_ w1163]
              tunnel: w1130 -> [_ w1162]
              tunnel: w1125 -> [_ w1157]
              frame False {
                n508 = Bundle By Name(cluster=T2 {"Level"=enum."L0_PAQ_10mil", "HigherLevel"=FALSE, "prev_pnt"=0, "last_pnt"=0} ("AverageAction"), "HigherLevel"=w1153) -> (w1152:T2)
              }
              frame True {
                n509 = in-place {
                  in-place-border: w1162 -> [w1170]
                  in-place-border: [w1173] -> w1160
                  in-place-border: [w1169] -> w1158
                  in-place-border: w1157 -> [w1168]
                  n510 = in-place-dvr #93(w1163) -> (w1172:refnum<class "PAQ-memory.lvclass">)  [unwired: 1 out]
                  n511 = in-place-match #94(w1164) -> (w1171:errorcluster)
                  n512 = call "PAQmem_WriteOne.vi"("Carry"=w1168, "error in (no error)"=w1171, "StoreDatagram"=w1170, "PAQ-memory in"=w1172) -> ("error out"=w1174:errorcluster, "Last"=w1173:i32, "Prev"=w1169:i32, "PAQ-memory out"=w1175:refnum<class "PAQ-memory.lvclass">)  [unwired: 4 in]
                  n513 = in-place-dvr #93(w1175) -> ()  [unwired: 2 out]
                  n514 = in-place-match #94(w1174) -> (w1167:errorcluster)
                }
                n515 = Bundle By Name(cluster=T2 {"Level"=enum."L0_PAQ_10mil", "HigherLevel"=FALSE, "prev_pnt"=0, "last_pnt"=0} ("AverageAction"), "HigherLevel"=w1157, "prev_pnt"=w1158, "Level"=typedef_Level."L3_PAQ_10min", "last_pnt"=w1160) -> (w1165:T2)
              }
            }
          }
          frame "L3_PAQ_10min" {
            w1194 = 3  # L3_10min
            w1196 = 2  # L2_1min
            # "T - 1 hr\nup to\nT + 1 hr"
            n516 = Unbundle By Name(w1202) -> ("Time"=w1210:dbl)
            n517 = Unbundle By Name(w1202) -> ("TagIndex"=w1206:i32[])
            n518 = Unbundle By Name(w1207) -> ("prev_pnt"=w1204:i32, "last_pnt"=w1203:i32)
            n519 = Subtract(x=w1210, y=1800.0) -> (x-y=w1208:dbl)
            n520 = Index Array(array=w1215, index #1=w1194, index #2=w1196) -> (element #1=w1198:refnum<data-value>, element #2=w1197:refnum<data-value>)
            n521 = Quotient & Remainder(x=w1208, y=3600.0) -> (floor(x/y)=w1191:dbl)  [unwired: 1 out]
            n522 = Bundle By Name(cluster=T4 {"TAGs"=[], "prev_pnt"=0, "last_pnt"=0} ("ChunkDefinition"), "TAGs"=w1206, "prev_pnt"=w1204, "last_pnt"=w1203) -> (w1199:T4)
            n523 = in-place {
              in-place-border: w1202 -> [w1250]
              in-place-border: [w1245] -> w1195
              in-place-border: w1199 -> [w1243]
              in-place-border: [w1241] -> w1193
              n524 = in-place-dvr #95(w1197) -> (w1253:refnum<class "PAQ-memory.lvclass">)  [unwired: 1 out]
              n525 = in-place-match #96(w1201) -> (w1252:errorcluster)
              n526 = call "PAQmem_ReadAverage.vi"("error in (no error)"=w1252, "ChunkDefinition"=w1243, "PAQ-memory in"=w1253) -> ("error out"=w1251:errorcluster, "Results"=w1254:T7, "PAQ-memory out"=w1244:refnum<class "PAQ-memory.lvclass">)  [unwired: 6 in]
              n527 = Unbundle By Name(w1254) -> ("data"=w1249:dbl[], "max"=w1248:dbl[], "min"=w1247:dbl[], "status"=w1246:u32[], "Time"=w1242:dbl)
              n528 = Not Equal To 0?(x=w1242) -> (x != 0?=w1241:bool)
              n529 = Bundle By Name(cluster=w1250, "data"=w1249, "max"=w1248, "min"=w1247, "status"=w1246, "Time"=w1242) -> (w1245:T3)
              n530 = in-place-dvr #95(w1244) -> ()  [unwired: 2 out]
              n531 = in-place-match #96(w1251) -> (w1200:errorcluster)
            }
            n532 = feedback #97() -> (w1192:dbl)  [unwired: 1 in]
            n533 = feedback-in #97(w1191) -> ()
            n534 = Not Equal?(x=w1191, y=w1192) -> (x != y?=w1190:bool)
            n535 = case shown="True" w1193 {
              selector: w1193 -> [w1218 _]
              tunnel: [w1220 w1232] -> w1216
              tunnel: [w1217 w1230] -> w1214
              tunnel: w1213 -> [w1221 w1224]
              tunnel: [w1221 w1224] -> w1212
              tunnel: w1200 -> [w1220 w1229]
              tunnel: w1198 -> [_ w1228]
              tunnel: w1195 -> [_ w1227]
              tunnel: w1190 -> [_ w1222]
              frame False {
                n536 = Bundle By Name(cluster=T2 {"Level"=enum."L0_PAQ_10mil", "HigherLevel"=FALSE, "prev_pnt"=0, "last_pnt"=0} ("AverageAction"), "HigherLevel"=w1218) -> (w1217:T2)
              }
              frame True {
                n537 = in-place {
                  in-place-border: w1227 -> [w1235]
                  in-place-border: [w1238] -> w1225
                  in-place-border: [w1234] -> w1223
                  in-place-border: w1222 -> [w1233]
                  n538 = in-place-dvr #98(w1228) -> (w1237:refnum<class "PAQ-memory.lvclass">)  [unwired: 1 out]
                  n539 = in-place-match #99(w1229) -> (w1236:errorcluster)
                  n540 = call "PAQmem_WriteOne.vi"("Carry"=w1233, "error in (no error)"=w1236, "StoreDatagram"=w1235, "PAQ-memory in"=w1237) -> ("error out"=w1239:errorcluster, "Last"=w1238:i32, "Prev"=w1234:i32, "PAQ-memory out"=w1240:refnum<class "PAQ-memory.lvclass">)  [unwired: 4 in]
                  n541 = in-place-dvr #98(w1240) -> ()  [unwired: 2 out]
                  n542 = in-place-match #99(w1239) -> (w1232:errorcluster)
                }
                n543 = Bundle By Name(cluster=T2 {"Level"=enum."L0_PAQ_10mil", "HigherLevel"=FALSE, "prev_pnt"=0, "last_pnt"=0} ("AverageAction"), "HigherLevel"=w1222, "prev_pnt"=w1223, "Level"=typedef_Level."L4_PAQ_2hr", "last_pnt"=w1225) -> (w1230:T2)
              }
            }
          }
          frame "L4_PAQ_2hr" {
            w1262 = 4  # L4_2hr
            w1264 = 3  # L3_10min
            # "check day passing"
            n544 = Unbundle By Name(w1270) -> ("Time"=w1261:dbl)
            n545 = Unbundle By Name(w1270) -> ("TagIndex"=w1274:i32[])
            n546 = Unbundle By Name(w1275) -> ("prev_pnt"=w1272:i32, "last_pnt"=w1271:i32)
            n547 = To Time Stamp(1:w1261) -> (0:w1260:timestamp)
            n548 = Format Into String(format string="%<%d-%m-%y>T", w1260) -> (resulting string=w1256:string)  [unwired: 2 in, 1 out]
            n549 = Index Array(array=w1279, index #1=w1262, index #2=w1264) -> (element #1=w1266:refnum<data-value>, element #2=w1265:refnum<data-value>)
            n550 = Bundle By Name(cluster=T4 {"TAGs"=[], "prev_pnt"=0, "last_pnt"=0} ("ChunkDefinition"), "TAGs"=w1274, "prev_pnt"=w1272, "last_pnt"=w1271) -> (w1267:T4)
            n551 = in-place {
              in-place-border: w1270 -> [w1314]
              in-place-border: [w1309] -> w1263
              in-place-border: w1267 -> [w1307]
              in-place-border: [w1305] -> w1258
              n552 = in-place-dvr #100(w1265) -> (w1317:refnum<class "PAQ-memory.lvclass">)  [unwired: 1 out]
              n553 = in-place-match #101(w1269) -> (w1316:errorcluster)
              n554 = call "PAQmem_ReadAverage.vi"("error in (no error)"=w1316, "ChunkDefinition"=w1307, "PAQ-memory in"=w1317) -> ("error out"=w1315:errorcluster, "Results"=w1318:T7, "PAQ-memory out"=w1308:refnum<class "PAQ-memory.lvclass">)  [unwired: 6 in]
              n555 = Unbundle By Name(w1318) -> ("data"=w1313:dbl[], "max"=w1312:dbl[], "min"=w1311:dbl[], "status"=w1310:u32[], "Time"=w1306:dbl)
              n556 = Not Equal To 0?(x=w1306) -> (x != 0?=w1305:bool)
              n557 = Bundle By Name(cluster=w1314, "data"=w1313, "max"=w1312, "min"=w1311, "status"=w1310, "Time"=w1306) -> (w1309:T3)
              n558 = in-place-dvr #100(w1308) -> ()  [unwired: 2 out]
              n559 = in-place-match #101(w1315) -> (w1268:errorcluster)
            }
            n560 = feedback #102() -> (w1257:string)  [unwired: 1 in]
            n561 = feedback-in #102(w1256) -> ()
            n562 = Not Equal?(x=w1256, y=w1257) -> (x != y?=w1255:bool)
            n563 = case "Averaged data valid?" shown="True" w1258 {
              selector: w1258 -> [w1282 _]
              tunnel: [w1284 w1296] -> w1280
              tunnel: [w1281 w1294] -> w1278
              tunnel: w1277 -> [w1285 w1286]
              tunnel: [w1285 w1286] -> w1276
              tunnel: w1268 -> [w1284 w1293]
              tunnel: w1266 -> [_ w1292]
              tunnel: w1263 -> [_ w1291]
              tunnel: w1255 -> [_ w1288]
              frame False {
                n564 = Bundle By Name(cluster=T2 {"Level"=enum."L0_PAQ_10mil", "HigherLevel"=FALSE, "prev_pnt"=0, "last_pnt"=0} ("AverageAction"), "HigherLevel"=w1282) -> (w1281:T2)
              }
              frame True {
                n565 = in-place {
                  in-place-border: w1291 -> [w1299]
                  in-place-border: [w1302] -> w1289
                  in-place-border: w1288 -> [w1298]
                  in-place-border: [w1297] -> w1287
                  n566 = in-place-dvr #103(w1292) -> (w1301:refnum<class "PAQ-memory.lvclass">)  [unwired: 1 out]
                  n567 = in-place-match #104(w1293) -> (w1300:errorcluster)
                  n568 = call "PAQmem_WriteOne.vi"("Carry"=w1298, "error in (no error)"=w1300, "StoreDatagram"=w1299, "PAQ-memory in"=w1301) -> ("error out"=w1303:errorcluster, "Last"=w1302:i32, "Prev"=w1297:i32, "PAQ-memory out"=w1304:refnum<class "PAQ-memory.lvclass">)  [unwired: 4 in]
                  n569 = in-place-dvr #103(w1304) -> ()  [unwired: 2 out]
                  n570 = in-place-match #104(w1303) -> (w1296:errorcluster)
                }
                n571 = Bundle By Name(cluster=T2 {"Level"=enum."L0_PAQ_10mil", "HigherLevel"=FALSE, "prev_pnt"=0, "last_pnt"=0} ("AverageAction"), "HigherLevel"=w1288, "prev_pnt"=w1287, "Level"=typedef_Level."L5_PAQ_1day", "last_pnt"=w1289) -> (w1294:T2)
              }
            }
          }
          frame "L5_PAQ_1day" {
            w1324 = 86400.0  # +1day
            w1328 = 5  # L5_1day
            w1330 = 4  # L4_2hr
            # "week sat/sun passing"
            n572 = Unbundle By Name(w1336) -> ("Time"=w1325:dbl)
            n573 = Unbundle By Name(w1336) -> ("TagIndex"=w1340:i32[])
            n574 = Unbundle By Name(w1341) -> ("prev_pnt"=w1338:i32, "last_pnt"=w1337:i32)
            n575 = Add(x=w1324, y=w1325) -> (x+y=w1323:dbl)
            n576 = Index Array(array=w1345, index #1=w1328, index #2=w1330) -> (element #1=w1332:refnum<data-value>, element #2=w1331:refnum<data-value>)
            n577 = Bundle By Name(cluster=T4 {"TAGs"=[], "prev_pnt"=0, "last_pnt"=0} ("ChunkDefinition"), "TAGs"=w1340, "prev_pnt"=w1338, "last_pnt"=w1337) -> (w1333:T4)
            n578 = To Time Stamp(1:w1323) -> (0:w1327:timestamp)
            n579 = in-place {
              in-place-border: w1336 -> [w1380]
              in-place-border: [w1375] -> w1329
              in-place-border: w1333 -> [w1373]
              in-place-border: [w1371] -> w1322
              n580 = in-place-dvr #105(w1331) -> (w1383:refnum<class "PAQ-memory.lvclass">)  [unwired: 1 out]
              n581 = in-place-match #106(w1335) -> (w1382:errorcluster)
              n582 = call "PAQmem_ReadAverage.vi"("error in (no error)"=w1382, "ChunkDefinition"=w1373, "PAQ-memory in"=w1383) -> ("error out"=w1381:errorcluster, "Results"=w1384:T7, "PAQ-memory out"=w1374:refnum<class "PAQ-memory.lvclass">)  [unwired: 6 in]
              n583 = Unbundle By Name(w1384) -> ("data"=w1379:dbl[], "max"=w1378:dbl[], "min"=w1377:dbl[], "status"=w1376:u32[], "Time"=w1372:dbl)
              n584 = Not Equal To 0?(x=w1372) -> (x != 0?=w1371:bool)
              n585 = Bundle By Name(cluster=w1380, "data"=w1379, "max"=w1378, "min"=w1377, "status"=w1376, "Time"=w1372) -> (w1375:T3)
              n586 = in-place-dvr #105(w1374) -> ()  [unwired: 2 out]
              n587 = in-place-match #106(w1381) -> (w1334:errorcluster)
            }
            n588 = Format Into String(format string="%<%W-%y>T", w1327) -> (resulting string=w1320:string)  [unwired: 2 in, 1 out]
            n589 = feedback #107() -> (w1321:string)  [unwired: 1 in]
            n590 = feedback-in #107(w1320) -> ()
            n591 = Not Equal?(x=w1320, y=w1321) -> (x != y?=w1319:bool)
            n592 = case "Averaged data valid?" shown="True" w1322 {
              selector: w1322 -> [w1348 _]
              tunnel: [w1351 w1362] -> w1346
              tunnel: [w1347 w1360] -> w1344
              tunnel: w1343 -> [w1350 w1354]
              tunnel: [w1350 w1354] -> w1342
              tunnel: w1334 -> [w1351 w1359]
              tunnel: w1332 -> [_ w1358]
              tunnel: w1329 -> [_ w1357]
              tunnel: w1319 -> [_ w1352]
              frame False {
                n593 = Bundle By Name(cluster=T2 {"Level"=enum."L0_PAQ_10mil", "HigherLevel"=FALSE, "prev_pnt"=0, "last_pnt"=0} ("AverageAction"), "HigherLevel"=w1348) -> (w1347:T2)
              }
              frame True {
                n594 = in-place {
                  in-place-border: w1357 -> [w1365]
                  in-place-border: [w1368] -> w1355
                  in-place-border: [w1364] -> w1353
                  in-place-border: w1352 -> [w1363]
                  n595 = in-place-dvr #108(w1358) -> (w1367:refnum<class "PAQ-memory.lvclass">)  [unwired: 1 out]
                  n596 = in-place-match #109(w1359) -> (w1366:errorcluster)
                  n597 = call "PAQmem_WriteOne.vi"("Carry"=w1363, "error in (no error)"=w1366, "StoreDatagram"=w1365, "PAQ-memory in"=w1367) -> ("error out"=w1369:errorcluster, "Last"=w1368:i32, "Prev"=w1364:i32, "PAQ-memory out"=w1370:refnum<class "PAQ-memory.lvclass">)  [unwired: 4 in]
                  n598 = in-place-dvr #108(w1370) -> ()  [unwired: 2 out]
                  n599 = in-place-match #109(w1369) -> (w1362:errorcluster)
                }
                n600 = Bundle By Name(cluster=T2 {"Level"=enum."L0_PAQ_10mil", "HigherLevel"=FALSE, "prev_pnt"=0, "last_pnt"=0} ("AverageAction"), "HigherLevel"=w1352, "prev_pnt"=w1353, "Level"=typedef_Level."L6_PAQ_1wk", "last_pnt"=w1355) -> (w1360:T2)
              }
            }
          }
          frame "L6_PAQ_1wk" {
            w1386 = 6  # L6_1wk
            w1388 = 5  # L5_1day
            n601 = Unbundle By Name(w1394) -> ("TagIndex"=w1398:i32[])
            n602 = Unbundle By Name(w1399) -> ("prev_pnt"=w1396:i32, "last_pnt"=w1395:i32)
            n603 = Index Array(array=w1403, index #1=w1386, index #2=w1388) -> (element #1=w1390:refnum<data-value>, element #2=w1389:refnum<data-value>)
            n604 = Bundle By Name(cluster=T4 {"TAGs"=[], "prev_pnt"=0, "last_pnt"=0} ("ChunkDefinition"), "TAGs"=w1398, "prev_pnt"=w1396, "last_pnt"=w1395) -> (w1391:T4)
            n605 = in-place {
              in-place-border: w1394 -> [w1433]
              in-place-border: [w1428] -> w1387
              in-place-border: w1391 -> [w1426]
              in-place-border: [w1424] -> w1385
              n606 = in-place-dvr #110(w1389) -> (w1436:refnum<class "PAQ-memory.lvclass">)  [unwired: 1 out]
              n607 = in-place-match #111(w1393) -> (w1435:errorcluster)
              n608 = call "PAQmem_ReadAverage.vi"("error in (no error)"=w1435, "ChunkDefinition"=w1426, "PAQ-memory in"=w1436) -> ("error out"=w1434:errorcluster, "Results"=w1437:T7, "PAQ-memory out"=w1427:refnum<class "PAQ-memory.lvclass">)  [unwired: 6 in]
              n609 = Unbundle By Name(w1437) -> ("data"=w1432:dbl[], "max"=w1431:dbl[], "min"=w1430:dbl[], "status"=w1429:u32[], "Time"=w1425:dbl)
              n610 = Not Equal To 0?(x=w1425) -> (x != 0?=w1424:bool)
              n611 = Bundle By Name(cluster=w1433, "data"=w1432, "max"=w1431, "min"=w1430, "status"=w1429, "Time"=w1425) -> (w1428:T3)
              n612 = in-place-dvr #110(w1427) -> ()  [unwired: 2 out]
              n613 = in-place-match #111(w1434) -> (w1392:errorcluster)
            }
            n614 = case "Averaged data valid?" shown="True" w1385 {
              selector: w1385 -> [w1406 _]
              tunnel: [w1408 w1417] -> w1404
              tunnel: [w1405 w1415] -> w1402
              tunnel: w1401 -> [w1409 w1411]
              tunnel: [w1409 w1411] -> w1400
              tunnel: w1392 -> [w1408 w1414]
              tunnel: w1390 -> [_ w1413]
              tunnel: w1387 -> [_ w1412]
              frame False {
                n615 = Bundle By Name(cluster=T2 {"Level"=enum."L0_PAQ_10mil", "HigherLevel"=FALSE, "prev_pnt"=0, "last_pnt"=0} ("AverageAction"), "HigherLevel"=w1406) -> (w1405:T2)
              }
              frame True {
                w1410 = FALSE
                n616 = in-place {
                  in-place-border: w1412 -> [w1419]
                  in-place-border: w1410 -> [w1418]
                  n617 = in-place-dvr #112(w1413) -> (w1421:refnum<class "PAQ-memory.lvclass">)  [unwired: 1 out]
                  n618 = in-place-match #113(w1414) -> (w1420:errorcluster)
                  n619 = call "PAQmem_WriteOne.vi"("Carry"=w1418, "error in (no error)"=w1420, "StoreDatagram"=w1419, "PAQ-memory in"=w1421) -> ("error out"=w1422:errorcluster, "PAQ-memory out"=w1423:refnum<class "PAQ-memory.lvclass">)  [unwired: 4 in, 2 out]
                  n620 = in-place-dvr #112(w1423) -> ()  [unwired: 2 out]
                  n621 = in-place-match #113(w1422) -> (w1417:errorcluster)
                }
                n622 = Bundle By Name(cluster=T2 {"Level"=enum."L0_PAQ_10mil", "HigherLevel"=FALSE, "prev_pnt"=0, "last_pnt"=0} ("AverageAction"), "HigherLevel"=w1410) -> (w1415:T2)
              }
            }
          }
          frame "L0_PAQ_10sec" {
            w1442 = 0  # L0_10sec
            # "T - 30 sec\nup to\nT + 30 sec"
            n623 = Unbundle By Name(w1444) -> ("Time"=w1449:dbl)
            n624 = Subtract(x=w1449, y=30.0) -> (x-y=w1447:dbl)
            n625 = Quotient & Remainder(x=w1447, y=60.0) -> (floor(x/y)=w1446:dbl)  [unwired: 1 out]
            n626 = Index Array(array=w1454, index=w1442) -> (element=w1453:refnum<data-value>)
            n627 = feedback #114() -> (w1445:dbl)  [unwired: 1 in]
            n628 = feedback-in #114(w1446) -> ()
            n629 = Not Equal?(x=w1446, y=w1445) -> (x != y?=w1439:bool)
            n630 = in-place {
              in-place-border: w1444 -> [w1462]
              in-place-border: [w1459] -> w1441
              in-place-border: w1439 -> [w1458]
              in-place-border: [w1457] -> w1438
              n631 = in-place-dvr #115(w1453) -> (w1464:refnum<class "PAQ-memory.lvclass">)  [unwired: 1 out]
              n632 = in-place-match #116(w1456) -> (w1461:errorcluster)
              n633 = call "PAQmem_WriteOne.vi"("Carry"=w1458, "error in (no error)"=w1461, "StoreDatagram"=w1462, "PAQ-memory in"=w1464) -> ("error out"=w1460:errorcluster, "Last"=w1459:i32, "Prev"=w1457:i32, "PAQ-memory out"=w1463:refnum<class "PAQ-memory.lvclass">)  [unwired: 4 in]
              n634 = in-place-dvr #115(w1463) -> ()  [unwired: 2 out]
              n635 = in-place-match #116(w1460) -> (w1455:errorcluster)
            }
            n636 = Bundle By Name(cluster=T2 {"Level"=enum."L0_PAQ_10mil", "HigherLevel"=FALSE, "prev_pnt"=0, "last_pnt"=0} ("AverageAction"), "HigherLevel"=w1439, "prev_pnt"=w1438, "last_pnt"=w1441, "Level"=typedef_Level."L1_PAQ_1min") -> (w1451:T2)
          }
          frame "L1_PAQ_1min" {
            w1469 = 1  # L1_1min
            w1471 = 0  # L0_10sec
            # "T - 5 min\nup to\nT + 5 min"
            n637 = Unbundle By Name(w1477) -> ("Time"=w1485:dbl)
            n638 = Unbundle By Name(w1477) -> ("TagIndex"=w1481:i32[])
            n639 = Unbundle By Name(w1482) -> ("prev_pnt"=w1479:i32, "last_pnt"=w1478:i32)
            n640 = Index Array(array=w1490, index #1=w1469, index #2=w1471) -> (element #1=w1473:refnum<data-value>, element #2=w1472:refnum<data-value>)
            n641 = Subtract(x=w1485, y=150.0) -> (x-y=w1483:dbl)
            n642 = Bundle By Name(cluster=T4 {"TAGs"=[], "prev_pnt"=0, "last_pnt"=0} ("ChunkDefinition"), "TAGs"=w1481, "prev_pnt"=w1479, "last_pnt"=w1478) -> (w1474:T4)
            n643 = Quotient & Remainder(x=w1483, y=300.0) -> (floor(x/y)=w1466:dbl)  [unwired: 1 out]
            n644 = in-place {
              in-place-border: w1477 -> [w1525]
              in-place-border: [w1520] -> w1470
              in-place-border: w1474 -> [w1518]
              in-place-border: [w1516] -> w1468
              n645 = in-place-dvr #117(w1472) -> (w1528:refnum<class "PAQ-memory.lvclass">)  [unwired: 1 out]
              n646 = in-place-match #118(w1476) -> (w1527:errorcluster)
              n647 = call "PAQmem_ReadAverage.vi"("error in (no error)"=w1527, "ChunkDefinition"=w1518, "PAQ-memory in"=w1528) -> ("error out"=w1526:errorcluster, "Results"=w1529:T7, "PAQ-memory out"=w1519:refnum<class "PAQ-memory.lvclass">)  [unwired: 6 in]
              n648 = Unbundle By Name(w1529) -> ("data"=w1524:dbl[], "max"=w1523:dbl[], "min"=w1522:dbl[], "status"=w1521:u32[], "Time"=w1517:dbl)
              n649 = Not Equal To 0?(x=w1517) -> (x != 0?=w1516:bool)
              n650 = Bundle By Name(cluster=w1525, "data"=w1524, "max"=w1523, "min"=w1522, "status"=w1521, "Time"=w1517) -> (w1520:T3)
              n651 = in-place-dvr #117(w1519) -> ()  [unwired: 2 out]
              n652 = in-place-match #118(w1526) -> (w1475:errorcluster)
            }
            n653 = feedback #119() -> (w1467:dbl)  [unwired: 1 in]
            n654 = feedback-in #119(w1466) -> ()
            n655 = Not Equal?(x=w1466, y=w1467) -> (x != y?=w1465:bool)
            n656 = case "Averaged data valid?" shown="True" w1468 {
              selector: w1468 -> [w1493 _]
              tunnel: [w1495 w1507] -> w1491
              tunnel: [w1492 w1505] -> w1489
              tunnel: w1488 -> [w1496 w1499]
              tunnel: [w1496 w1499] -> w1487
              tunnel: w1475 -> [w1495 w1504]
              tunnel: w1473 -> [_ w1503]
              tunnel: w1470 -> [_ w1502]
              tunnel: w1465 -> [_ w1497]
              frame False {
                n657 = Bundle By Name(cluster=T2 {"Level"=enum."L0_PAQ_10mil", "HigherLevel"=FALSE, "prev_pnt"=0, "last_pnt"=0} ("AverageAction"), "HigherLevel"=w1493) -> (w1492:T2)
              }
              frame True {
                n658 = in-place {
                  in-place-border: w1502 -> [w1510]
                  in-place-border: [w1513] -> w1500
                  in-place-border: [w1509] -> w1498
                  in-place-border: w1497 -> [w1508]
                  n659 = in-place-dvr #120(w1503) -> (w1512:refnum<class "PAQ-memory.lvclass">)  [unwired: 1 out]
                  n660 = in-place-match #121(w1504) -> (w1511:errorcluster)
                  n661 = call "PAQmem_WriteOne.vi"("Carry"=w1508, "error in (no error)"=w1511, "StoreDatagram"=w1510, "PAQ-memory in"=w1512) -> ("error out"=w1514:errorcluster, "Last"=w1513:i32, "Prev"=w1509:i32, "PAQ-memory out"=w1515:refnum<class "PAQ-memory.lvclass">)  [unwired: 4 in]
                  n662 = in-place-dvr #120(w1515) -> ()  [unwired: 2 out]
                  n663 = in-place-match #121(w1514) -> (w1507:errorcluster)
                }
                n664 = Bundle By Name(cluster=T2 {"Level"=enum."L0_PAQ_10mil", "HigherLevel"=FALSE, "prev_pnt"=0, "last_pnt"=0} ("AverageAction"), "HigherLevel"=w1497, "prev_pnt"=w1498, "Level"=typedef_Level."L2_PAQ_10min", "last_pnt"=w1500) -> (w1505:T2)
              }
            }
          }
          frame "L2_PAQ_10min" {
            w1534 = 2  # L2_10min
            w1536 = 1  # L1_1min
            # "T - 1 hr\nup to\nT + 1 hr"
            n665 = Unbundle By Name(w1542) -> ("Time"=w1550:dbl)
            n666 = Unbundle By Name(w1542) -> ("TagIndex"=w1546:i32[])
            n667 = Unbundle By Name(w1547) -> ("prev_pnt"=w1544:i32, "last_pnt"=w1543:i32)
            n668 = Index Array(array=w1555, index #1=w1534, index #2=w1536) -> (element #1=w1538:refnum<data-value>, element #2=w1537:refnum<data-value>)
            n669 = Subtract(x=w1550, y=1800.0) -> (x-y=w1548:dbl)
            n670 = Bundle By Name(cluster=T4 {"TAGs"=[], "prev_pnt"=0, "last_pnt"=0} ("ChunkDefinition"), "TAGs"=w1546, "prev_pnt"=w1544, "last_pnt"=w1543) -> (w1539:T4)
            n671 = Quotient & Remainder(x=w1548, y=3600.0) -> (floor(x/y)=w1531:dbl)  [unwired: 1 out]
            n672 = in-place {
              in-place-border: w1542 -> [w1590]
              in-place-border: [w1585] -> w1535
              in-place-border: w1539 -> [w1583]
              in-place-border: [w1581] -> w1533
              n673 = in-place-dvr #122(w1537) -> (w1593:refnum<class "PAQ-memory.lvclass">)  [unwired: 1 out]
              n674 = in-place-match #123(w1541) -> (w1592:errorcluster)
              n675 = call "PAQmem_ReadAverage.vi"("error in (no error)"=w1592, "ChunkDefinition"=w1583, "PAQ-memory in"=w1593) -> ("error out"=w1591:errorcluster, "Results"=w1594:T7, "PAQ-memory out"=w1584:refnum<class "PAQ-memory.lvclass">)  [unwired: 6 in]
              n676 = Unbundle By Name(w1594) -> ("data"=w1589:dbl[], "max"=w1588:dbl[], "min"=w1587:dbl[], "status"=w1586:u32[], "Time"=w1582:dbl)
              n677 = Not Equal To 0?(x=w1582) -> (x != 0?=w1581:bool)
              n678 = Bundle By Name(cluster=w1590, "data"=w1589, "max"=w1588, "min"=w1587, "status"=w1586, "Time"=w1582) -> (w1585:T3)
              n679 = in-place-dvr #122(w1584) -> ()  [unwired: 2 out]
              n680 = in-place-match #123(w1591) -> (w1540:errorcluster)
            }
            n681 = feedback #124() -> (w1532:dbl)  [unwired: 1 in]
            n682 = feedback-in #124(w1531) -> ()
            n683 = Not Equal?(x=w1531, y=w1532) -> (x != y?=w1530:bool)
            n684 = case "Averaged data valid?" shown="True" w1533 {
              selector: w1533 -> [w1559 _]
              tunnel: [w1558 w1572] -> w1556
              tunnel: [w1560 w1570] -> w1554
              tunnel: w1553 -> [w1557 w1562]
              tunnel: [w1557 w1562] -> w1552
              tunnel: w1540 -> [w1558 w1569]
              tunnel: w1538 -> [_ w1568]
              tunnel: w1535 -> [_ w1567]
              tunnel: w1530 -> [_ w1563]
              frame False {
                n685 = Bundle By Name(cluster=T2 {"Level"=enum."L0_PAQ_10mil", "HigherLevel"=FALSE, "prev_pnt"=0, "last_pnt"=0} ("AverageAction"), "HigherLevel"=w1559) -> (w1560:T2)
              }
              frame True {
                n686 = in-place {
                  in-place-border: w1567 -> [w1575]
                  in-place-border: [w1578] -> w1565
                  in-place-border: [w1574] -> w1564
                  in-place-border: w1563 -> [w1573]
                  n687 = in-place-dvr #125(w1568) -> (w1577:refnum<class "PAQ-memory.lvclass">)  [unwired: 1 out]
                  n688 = in-place-match #126(w1569) -> (w1576:errorcluster)
                  n689 = call "PAQmem_WriteOne.vi"("Carry"=w1573, "error in (no error)"=w1576, "StoreDatagram"=w1575, "PAQ-memory in"=w1577) -> ("error out"=w1579:errorcluster, "Last"=w1578:i32, "Prev"=w1574:i32, "PAQ-memory out"=w1580:refnum<class "PAQ-memory.lvclass">)  [unwired: 4 in]
                  n690 = in-place-dvr #125(w1580) -> ()  [unwired: 2 out]
                  n691 = in-place-match #126(w1579) -> (w1572:errorcluster)
                }
                n692 = Bundle By Name(cluster=T2 {"Level"=enum."L0_PAQ_10mil", "HigherLevel"=FALSE, "prev_pnt"=0, "last_pnt"=0} ("AverageAction"), "HigherLevel"=w1563, "prev_pnt"=w1564, "Level"=typedef_Level."L3_PAQ_2hr", "last_pnt"=w1565) -> (w1570:T2)
              }
            }
          }
          frame "L3_PAQ_2hr" {
            w1602 = 3  # L3_2hr
            w1604 = 2  # L2_10min
            # "check day passing"
            n693 = Unbundle By Name(w1610) -> ("TagIndex"=w1614:i32[])
            n694 = Unbundle By Name(w1615) -> ("prev_pnt"=w1612:i32, "last_pnt"=w1611:i32)
            n695 = Unbundle By Name(w1610) -> ("Time"=w1601:dbl)
            n696 = To Time Stamp(1:w1601) -> (0:w1600:timestamp)
            n697 = Index Array(array=w1619, index #1=w1602, index #2=w1604) -> (element #1=w1606:refnum<data-value>, element #2=w1605:refnum<data-value>)
            n698 = Format Into String(format string="%<%d-%m-%y>T", w1600) -> (resulting string=w1596:string)  [unwired: 2 in, 1 out]
            n699 = Bundle By Name(cluster=T4 {"TAGs"=[], "prev_pnt"=0, "last_pnt"=0} ("ChunkDefinition"), "TAGs"=w1614, "prev_pnt"=w1612, "last_pnt"=w1611) -> (w1607:T4)
            n700 = in-place {
              in-place-border: w1610 -> [w1654]
              in-place-border: [w1649] -> w1603
              in-place-border: w1607 -> [w1647]
              in-place-border: [w1645] -> w1598
              n701 = in-place-dvr #127(w1605) -> (w1657:refnum<class "PAQ-memory.lvclass">)  [unwired: 1 out]
              n702 = in-place-match #128(w1609) -> (w1656:errorcluster)
              n703 = call "PAQmem_ReadAverage.vi"("error in (no error)"=w1656, "ChunkDefinition"=w1647, "PAQ-memory in"=w1657) -> ("error out"=w1655:errorcluster, "Results"=w1658:T7, "PAQ-memory out"=w1648:refnum<class "PAQ-memory.lvclass">)  [unwired: 6 in]
              n704 = Unbundle By Name(w1658) -> ("data"=w1653:dbl[], "max"=w1652:dbl[], "min"=w1651:dbl[], "status"=w1650:u32[], "Time"=w1646:dbl)
              n705 = Not Equal To 0?(x=w1646) -> (x != 0?=w1645:bool)
              n706 = Bundle By Name(cluster=w1654, "data"=w1653, "max"=w1652, "min"=w1651, "status"=w1650, "Time"=w1646) -> (w1649:T3)
              n707 = in-place-dvr #127(w1648) -> ()  [unwired: 2 out]
              n708 = in-place-match #128(w1655) -> (w1608:errorcluster)
            }
            n709 = feedback #129() -> (w1597:string)  [unwired: 1 in]
            n710 = feedback-in #129(w1596) -> ()
            n711 = Not Equal?(x=w1596, y=w1597) -> (x != y?=w1595:bool)
            n712 = case "Averaged data valid?" shown="True" w1598 {
              selector: w1598 -> [w1623 _]
              tunnel: [w1625 w1636] -> w1620
              tunnel: [w1622 w1634] -> w1618
              tunnel: w1617 -> [w1621 w1628]
              tunnel: [w1621 w1628] -> w1616
              tunnel: w1608 -> [w1625 w1633]
              tunnel: w1606 -> [_ w1632]
              tunnel: w1603 -> [_ w1631]
              tunnel: w1595 -> [_ w1627]
              frame False {
                n713 = Bundle By Name(cluster=T2 {"Level"=enum."L0_PAQ_10mil", "HigherLevel"=FALSE, "prev_pnt"=0, "last_pnt"=0} ("AverageAction"), "HigherLevel"=w1623) -> (w1622:T2)
              }
              frame True {
                n714 = in-place {
                  in-place-border: w1631 -> [w1639]
                  in-place-border: [w1642] -> w1629
                  in-place-border: w1627 -> [w1638]
                  in-place-border: [w1637] -> w1626
                  n715 = in-place-dvr #130(w1632) -> (w1641:refnum<class "PAQ-memory.lvclass">)  [unwired: 1 out]
                  n716 = in-place-match #131(w1633) -> (w1640:errorcluster)
                  n717 = call "PAQmem_WriteOne.vi"("Carry"=w1638, "error in (no error)"=w1640, "StoreDatagram"=w1639, "PAQ-memory in"=w1641) -> ("error out"=w1643:errorcluster, "Last"=w1642:i32, "Prev"=w1637:i32, "PAQ-memory out"=w1644:refnum<class "PAQ-memory.lvclass">)  [unwired: 4 in]
                  n718 = in-place-dvr #130(w1644) -> ()  [unwired: 2 out]
                  n719 = in-place-match #131(w1643) -> (w1636:errorcluster)
                }
                n720 = Bundle By Name(cluster=T2 {"Level"=enum."L0_PAQ_10mil", "HigherLevel"=FALSE, "prev_pnt"=0, "last_pnt"=0} ("AverageAction"), "HigherLevel"=w1627, "prev_pnt"=w1626, "Level"=typedef_Level."L4_PAQ_1day", "last_pnt"=w1629) -> (w1634:T2)
              }
            }
          }
          frame "L4_PAQ_1day" {
            w1664 = 86400.0  # +1day
            w1668 = 4  # L4_1day
            w1670 = 3  # L3_2hr
            # "week sat/sun passing"
            n721 = Unbundle By Name(w1676) -> ("TagIndex"=w1680:i32[])
            n722 = Unbundle By Name(w1681) -> ("prev_pnt"=w1678:i32, "last_pnt"=w1677:i32)
            n723 = Unbundle By Name(w1676) -> ("Time"=w1665:dbl)
            n724 = Add(x=w1664, y=w1665) -> (x+y=w1663:dbl)
            n725 = Index Array(array=w1685, index #1=w1668, index #2=w1670) -> (element #1=w1672:refnum<data-value>, element #2=w1671:refnum<data-value>)
            n726 = To Time Stamp(1:w1663) -> (0:w1667:timestamp)
            n727 = Bundle By Name(cluster=T4 {"TAGs"=[], "prev_pnt"=0, "last_pnt"=0} ("ChunkDefinition"), "TAGs"=w1680, "prev_pnt"=w1678, "last_pnt"=w1677) -> (w1673:T4)
            n728 = Format Into String(format string="%<%W-%y>T", w1667) -> (resulting string=w1660:string)  [unwired: 2 in, 1 out]
            n729 = in-place {
              in-place-border: w1676 -> [w1720]
              in-place-border: [w1715] -> w1669
              in-place-border: w1673 -> [w1713]
              in-place-border: [w1711] -> w1662
              n730 = in-place-dvr #132(w1671) -> (w1723:refnum<class "PAQ-memory.lvclass">)  [unwired: 1 out]
              n731 = in-place-match #133(w1675) -> (w1722:errorcluster)
              n732 = call "PAQmem_ReadAverage.vi"("error in (no error)"=w1722, "ChunkDefinition"=w1713, "PAQ-memory in"=w1723) -> ("error out"=w1721:errorcluster, "Results"=w1724:T7, "PAQ-memory out"=w1714:refnum<class "PAQ-memory.lvclass">)  [unwired: 6 in]
              n733 = Unbundle By Name(w1724) -> ("data"=w1719:dbl[], "max"=w1718:dbl[], "min"=w1717:dbl[], "status"=w1716:u32[], "Time"=w1712:dbl)
              n734 = Not Equal To 0?(x=w1712) -> (x != 0?=w1711:bool)
              n735 = Bundle By Name(cluster=w1720, "data"=w1719, "max"=w1718, "min"=w1717, "status"=w1716, "Time"=w1712) -> (w1715:T3)
              n736 = in-place-dvr #132(w1714) -> ()  [unwired: 2 out]
              n737 = in-place-match #133(w1721) -> (w1674:errorcluster)
            }
            n738 = feedback #134() -> (w1661:string)  [unwired: 1 in]
            n739 = feedback-in #134(w1660) -> ()
            n740 = Not Equal?(x=w1660, y=w1661) -> (x != y?=w1659:bool)
            n741 = case "Averaged data valid?" shown="True" w1662 {
              selector: w1662 -> [w1688 _]
              tunnel: [w1690 w1702] -> w1686
              tunnel: [w1687 w1700] -> w1684
              tunnel: w1683 -> [w1691 w1692]
              tunnel: [w1691 w1692] -> w1682
              tunnel: w1674 -> [w1690 w1699]
              tunnel: w1672 -> [_ w1698]
              tunnel: w1669 -> [_ w1697]
              tunnel: w1659 -> [_ w1693]
              frame False {
                n742 = Bundle By Name(cluster=T2 {"Level"=enum."L0_PAQ_10mil", "HigherLevel"=FALSE, "prev_pnt"=0, "last_pnt"=0} ("AverageAction"), "HigherLevel"=w1688) -> (w1687:T2)
              }
              frame True {
                n743 = in-place {
                  in-place-border: w1697 -> [w1705]
                  in-place-border: [w1708] -> w1695
                  in-place-border: [w1704] -> w1694
                  in-place-border: w1693 -> [w1703]
                  n744 = in-place-dvr #135(w1698) -> (w1707:refnum<class "PAQ-memory.lvclass">)  [unwired: 1 out]
                  n745 = in-place-match #136(w1699) -> (w1706:errorcluster)
                  n746 = call "PAQmem_WriteOne.vi"("Carry"=w1703, "error in (no error)"=w1706, "StoreDatagram"=w1705, "PAQ-memory in"=w1707) -> ("error out"=w1709:errorcluster, "Last"=w1708:i32, "Prev"=w1704:i32, "PAQ-memory out"=w1710:refnum<class "PAQ-memory.lvclass">)  [unwired: 4 in]
                  n747 = in-place-dvr #135(w1710) -> ()  [unwired: 2 out]
                  n748 = in-place-match #136(w1709) -> (w1702:errorcluster)
                }
                n749 = Bundle By Name(cluster=T2 {"Level"=enum."L0_PAQ_10mil", "HigherLevel"=FALSE, "prev_pnt"=0, "last_pnt"=0} ("AverageAction"), "HigherLevel"=w1693, "prev_pnt"=w1694, "Level"=typedef_Level."L5_PAQ_1wk", "last_pnt"=w1695) -> (w1700:T2)
              }
            }
          }
          frame "L5_PAQ_1wk" {
            w1726 = 5  # L5_1wk
            w1728 = 4  # L4_1day
            n750 = Unbundle By Name(w1734) -> ("TagIndex"=w1738:i32[])
            n751 = Unbundle By Name(w1739) -> ("prev_pnt"=w1736:i32, "last_pnt"=w1735:i32)
            n752 = Index Array(array=w1743, index #1=w1726, index #2=w1728) -> (element #1=w1730:refnum<data-value>, element #2=w1729:refnum<data-value>)
            n753 = Bundle By Name(cluster=T4 {"TAGs"=[], "prev_pnt"=0, "last_pnt"=0} ("ChunkDefinition"), "TAGs"=w1738, "prev_pnt"=w1736, "last_pnt"=w1735) -> (w1731:T4)
            n754 = in-place {
              in-place-border: w1734 -> [w1773]
              in-place-border: [w1768] -> w1727
              in-place-border: w1731 -> [w1766]
              in-place-border: [w1764] -> w1725
              n755 = in-place-dvr #137(w1729) -> (w1776:refnum<class "PAQ-memory.lvclass">)  [unwired: 1 out]
              n756 = in-place-match #138(w1733) -> (w1775:errorcluster)
              n757 = call "PAQmem_ReadAverage.vi"("error in (no error)"=w1775, "ChunkDefinition"=w1766, "PAQ-memory in"=w1776) -> ("error out"=w1774:errorcluster, "Results"=w1777:T7, "PAQ-memory out"=w1767:refnum<class "PAQ-memory.lvclass">)  [unwired: 6 in]
              n758 = Unbundle By Name(w1777) -> ("data"=w1772:dbl[], "max"=w1771:dbl[], "min"=w1770:dbl[], "status"=w1769:u32[], "Time"=w1765:dbl)
              n759 = Not Equal To 0?(x=w1765) -> (x != 0?=w1764:bool)
              n760 = Bundle By Name(cluster=w1773, "data"=w1772, "max"=w1771, "min"=w1770, "status"=w1769, "Time"=w1765) -> (w1768:T3)
              n761 = in-place-dvr #137(w1767) -> ()  [unwired: 2 out]
              n762 = in-place-match #138(w1774) -> (w1732:errorcluster)
            }
            n763 = case "Averaged data valid?" shown="True" w1725 {
              selector: w1725 -> [w1747 _]
              tunnel: [w1746 w1757] -> w1744
              tunnel: [w1745 w1755] -> w1742
              tunnel: w1741 -> [w1749 w1751]
              tunnel: [w1749 w1751] -> w1740
              tunnel: w1732 -> [w1746 w1754]
              tunnel: w1730 -> [_ w1753]
              tunnel: w1727 -> [_ w1752]
              frame False {
                n764 = Bundle By Name(cluster=T2 {"Level"=enum."L0_PAQ_10mil", "HigherLevel"=FALSE, "prev_pnt"=0, "last_pnt"=0} ("AverageAction"), "HigherLevel"=w1747) -> (w1745:T2)
              }
              frame True {
                w1750 = FALSE
                n765 = in-place {
                  in-place-border: w1752 -> [w1759]
                  in-place-border: w1750 -> [w1758]
                  n766 = in-place-dvr #139(w1753) -> (w1761:refnum<class "PAQ-memory.lvclass">)  [unwired: 1 out]
                  n767 = in-place-match #140(w1754) -> (w1760:errorcluster)
                  n768 = call "PAQmem_WriteOne.vi"("Carry"=w1758, "error in (no error)"=w1760, "StoreDatagram"=w1759, "PAQ-memory in"=w1761) -> ("error out"=w1762:errorcluster, "PAQ-memory out"=w1763:refnum<class "PAQ-memory.lvclass">)  [unwired: 4 in, 2 out]
                  n769 = in-place-dvr #139(w1763) -> ()  [unwired: 2 out]
                  n770 = in-place-match #140(w1762) -> (w1757:errorcluster)
                }
                n771 = Bundle By Name(cluster=T2 {"Level"=enum."L0_PAQ_10mil", "HigherLevel"=FALSE, "prev_pnt"=0, "last_pnt"=0} ("AverageAction"), "HigherLevel"=w1750) -> (w1755:T2)
              }
            }
          }
        }
        n772 = in-place-dvr #1(w25) -> ()  [unwired: 2 out]
        n773 = in-place-match #2(w23) -> (w15:errorcluster)
      }
    }
    frame Error {
    }
  }
  "error out" <- w7
  "FAMM out" <- w5
  "Next_Level" <- w3
